vi "XW_Analysis_PN.vi"() -> (5 "Plug in titles":string[](array[string]), 7 "Plug in values":string[](array[string]))   [LabVIEW 2010]
uses:
  Controls/Save_Data.ctl
  Globals/Meas_global.vi
  Globals/Constants_global.vi
  Globals/Plug_in_data_global.vi
  <vilib>/Analysis/2dsp.llb/1D Auto Correlation (DBL).vi
  <vilib>/Analysis/2dsp.llb/1D Cross Correlation (DBL).vi
  Globals/Dynamic_call_global.ph.vi
  Controls/Inst_type.ctl
  <vilib>/Analysis/NI_AALPro.lvlib
panel:
  in  "Base output dir.":path=path "E:/TEST DUMP/QA test"
  in  "Instr. trav. pos index":i32=1 caption="Max moment order (n)"
  out "2nd comp.":string="v"
  out "DWT V":dbl[][](array[numeric])
  out "DWT U":dbl[][](array[numeric])
  out "Moment labels":string="u2\tu3\tu4\tv2\tv3\tv4\tu1v1\tu1v2\tu1v3\tu2v1\tu2v2\tu2v3\tu3v1\tu3v2\tu3v3\t"
  out "Moments":dbl[](array[numeric])=[1722182.8833231796, -3886.3484720409974, 2673329.388548149, 486662.5789464589, 30099.864061399367, 267894.77768629417, -362874.60480439797, -27342.46465798058, -171575.27046364895, 45307.846153853105, 346204.8570758366, 46417.28583948715, -555849.2877538406, -57883.486515684475, -276668.57969799754]
  in  "Max moment order (n)":i32=4
  in  "Psi pull-out search strings":string[](array[string])=["Psi 1:Average:Deg", "Psi 2:Average:Deg", "Psi 1:Max:Deg", "Psi 1:Min:Deg", "Psi 2:Max:Deg", "Psi 2:Min:Deg"]
  out "PwrSpec of UV":dbl[](array[numeric])
  out "AutoCovariance of UV":dbl[](array[numeric])
  out "Stats":dbl[][](array[numeric])=[[6.575279786237041, 9.737852813428246, 3.6304504106485544], [-0.05245759359759979, 2.477699101876975, -2.6510166405627658], [-0.4658815564167448, 17.436881271482232, -18.021292714723874]]
  in  "Use existing temp. block files":bool
  out "1D PDF UV":dbl[](array[numeric])=[0.0006999999999999999, 0.0012000000000000001, 0.0023, 0.009600000000000001, 0.021700000000000004, 0.04720000000000004, 0.1258000000000002, 0.3432, 0.8350999999999993, 1.9702000000000002, 4.395100000000001, 9.119700000000003, 17.268799999999995, 28.958799999999968, 41.936999999999976, 50.98729999999999, 50.53780000000002, 40.73420000000001, 26.46519999999999, 14.681399999999996, 6.8766, 2.8771999999999998, 1.1358999999999995, 0.4279000000000001, 0.14960000000000012, 0.055700000000000034, 0.021399999999999995, 0.008799999999999999, 0.0029000000000000007, 0.0009000000000000001, 0.0005, 0.0002]
  out "Axis UV":dbl[](array[numeric])=[-17.001377181562503, -15.8933092446875, -14.785241307812502, -13.677173370937501, -12.569105434062502, -11.461037497187501, -10.352969560312502, -9.244901623437501, -8.136833686562502, -7.028765749687502, -5.920697812812501, -4.8126298759375015, -3.7045619390625024, -2.5964940021875025, -1.4884260653125017, -0.3803581284375017, 0.7277098084374973, 1.8357777453124964, 2.943845682187497, 4.051913619062498, 5.159981555937497, 6.268049492812498, 7.376117429687499, 8.484185366562498, 9.592253303437497, 10.700321240312496, 11.808389177187497, 12.916457114062498, 14.024525050937497, 15.132592987812497, 16.240660924687496, 17.348728861562495] format="%0.2f"
  out "CrossPhaseSpec":dbl[](array[numeric])
  out "CrossPwrSpec":dbl[](array[numeric])
  out "df XPS":dbl=2.0 format="%0.2f"
  out "df APS":dbl=2.0 format="%0.2f"
  out "PwrSpec of U":dbl[](array[numeric])
  out "PwrSpec of V":dbl[](array[numeric])
  out "1D PDF V":dbl[](array[numeric])=[0.0002, 0.0002, 0.0007, 0.0023, 0.007300000000000003, 0.020099999999999996, 0.051100000000000007, 0.1565000000000002, 0.4621, 1.290799999999999, 3.148200000000002, 7.410600000000004, 15.145800000000001, 26.785999999999987, 39.79410000000002, 48.68330000000001, 48.59359999999999, 40.41779999999998, 28.99750000000001, 18.314799999999995, 10.619500000000002, 5.535599999999994, 2.625100000000002, 1.1498999999999997, 0.4730000000000003, 0.19190000000000013, 0.07570000000000006, 0.02819999999999999, 0.012799999999999997, 0.0037999999999999996, 0.0011, 0.00039999999999999996]
  out "Axis V":dbl[](array[numeric])=[-2.5184228665625, -2.3581504996875, -2.1978781328125, -2.0376057659375, -1.8773333990624999, -1.7170610321875, -1.5567886653124998, -1.3965162984375, -1.2362439315624998, -1.0759715646874999, -0.9156991978124999, -0.7554268309374998, -0.5951544640624997, -0.4348820971874998, -0.2746097303124999, -0.11433736343749978, 0.045935003437500344, 0.20620737031250047, 0.3664797371875004, 0.5267521040625003, 0.6870244709375004, 0.8472968378125003, 1.0075692046875002, 1.1678415715625003, 1.3281139384375003, 1.4883863053125004, 1.6486586721875005, 1.8089310390625002, 1.9692034059375003, 2.1294757728125004, 2.2897481396875006, 2.4500205065625007] format="%0.2f"
  out "Axis U":dbl[](array[numeric])=[-2.8494012174999996, -2.6585448925, -2.4676885674999998, -2.2768322425, -2.0859759175, -1.8951195925, -1.7042632674999998, -1.5134069424999999, -1.3225506175, -1.1316942925, -0.9408379675, -0.7499816424999999, -0.5591253174999997, -0.3682689924999998, -0.17741266749999984, 0.013443657500000095, 0.20429998250000003, 0.39515630749999997, 0.5860126324999999, 0.7768689574999998, 0.9677252825, 1.1585816075, 1.3494379324999999, 1.5402942575000003, 1.7311505825000002, 1.9220069075000001, 2.1128632325, 2.3037195575, 2.4945758825, 2.6854322075, 2.8762885325, 3.0671448574999998] format="%0.2f"
  out "1D PDF U":dbl[](array[numeric])=[0.0013000000000000002, 0.013600000000000001, 0.05110000000000003, 0.17249999999999993, 0.5014000000000004, 1.1012999999999988, 2.3825999999999983, 4.467200000000003, 7.386500000000001, 10.810400000000008, 14.8375, 19.03289999999999, 22.8511, 25.997799999999998, 27.798999999999992, 28.409600000000005, 27.990199999999987, 25.913499999999978, 22.712899999999976, 18.6365, 14.244500000000011, 10.149700000000005, 6.762300000000002, 3.9479000000000006, 2.1491000000000002, 1.0349999999999995, 0.39960000000000007, 0.16249999999999995, 0.04880000000000002, 0.0188, 0.012000000000000002, 0.0009]
  in  "XCovar algorithm":enum32{"direct", "frequency domain"}(ring)=enum."frequency domain"
  out "CrossCovariance":dbl[](array[numeric])
  in  "Non-dimensionalise covariance / spectra":bool=TRUE
  in  "Covariance normalisation":enum32{"none", "unbiased", "biased"}(ring)
  out "AutoCovariance of V":dbl[](array[numeric])
  out "AutoCovariance of U":dbl[](array[numeric])
  out "Post-Proc Block No.":i32=300
  in  "Interactive graph":bool
  in  "Mean shift PDFs":bool=TRUE
  in  "Nbins V":i32=32
  in  "Nbins U":i32=32
  in  "PDF (T) or Hist (F)":bool=TRUE
  out "VbinWidth":dbl=5.1287157400000005
  out "UbinWidth":dbl=6.1074024
  out "V bin centre vals.":dbl[](array[numeric])=[-0.03420117999999972]
  out "U bin centre vals.":dbl[](array[numeric])=[0.10887182000000006]
  out "2D PDF":dbl[][](array[numeric])=[[0.031925288878877155]]
  out "Quadrant probability":dbl[](array[numeric])=[0.18550766666666668, 0.31311866666666643, 0.3267083333333332, 0.17466533333333317]
  in  "Analysis":i32[](listbox)=[0, 1, 2, 4, 5, 6, 7]
  in  "format string":string="%.16f"
  in  "Instr. indices":i32[](array[numeric])=[1, 2]
  in  "Mode":enum16{"Spectra", "Autocorrelation"}(ring)
  in  "Separation Character":string="\t"
  in  "Precision":i16=16
  out "Ch names":string[](array[string])
  out "Output Directory":path=path "E:/TEST DUMP/QA test"
  in  "File":T1=enum."Save Data"
  # "You must have just these two indicators on the connector pane of the vi"
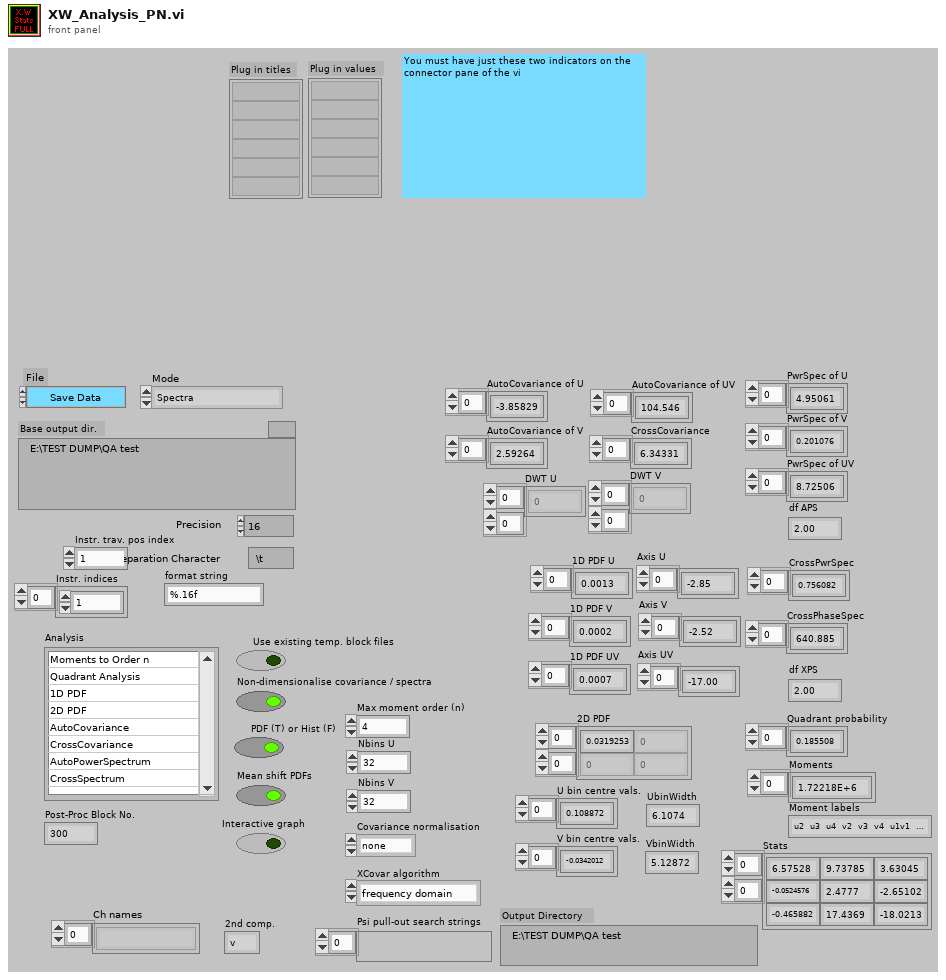
[diagram p1: front panel]
types:
  T1 = typedef "Save_Data.ctl" = enum16{"Save No Data", "Save Data"}
  T2 = typedef "Inst_type.ctl" = enum16{"Propeller anemometer", "Raw voltage", "Pressure Transducer", "Pitot-static tube", "Preston tube", "Hot wire", "Cross wire 1", "Cross wire 2", "Generic Linear", "Generic Polynomial", "Generic BackPoly", "Fast FID", "Thermocouple", "Cold wire", "Pulsed Wire", "LDA Vel", "LDA Tran time", "LDA Arr time"}
  T3 = enum32{"existing file", "new file", "new or existing file", "existing dir", "new dir", "new or existing dir", "existing file (use LLBs)", "new file (use LLBs)", "new or existing file (use LLBs)", "new or existing file or directory (use LLBs)"}
  T4 = cluster{"Name":string, "X":dbl, "Y":dbl, "Z":dbl}[]
  T5 = cluster{"Name":string, "X":dbl, "Y":dbl, "Z":dbl}
  T6 = typedef "Analysis_info_cluster.ctl" = cluster{"Colour":u32, "Inst type":T2, "Inst name":string, "Symbol":string, "Code name":string, "Extra Info":string, "Inst Array":T7, "Index":i32, "Voltage Index":i32, "Extra Titles":string[], "Extra Values":string[]}
  T7 = typedef "Instrument_Array.ctl" = enum16{"PWA", "LDA", "Analogue"}
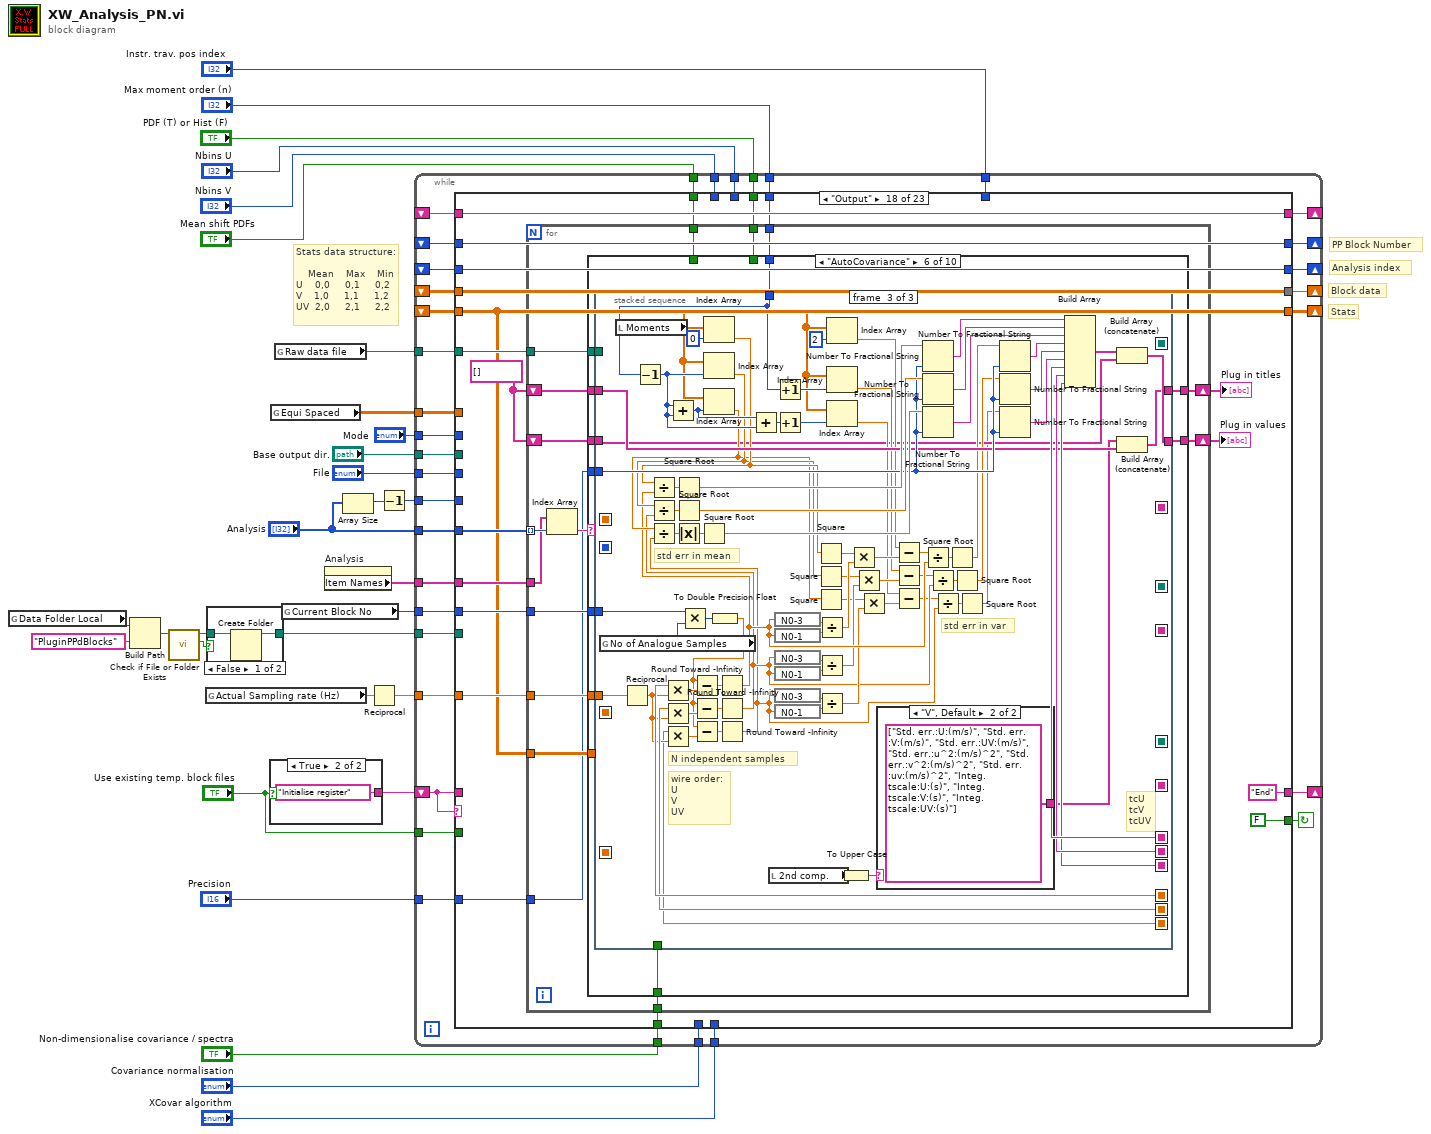
[diagram p0: block diagram]
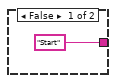
[diagram p3: hidden frame]
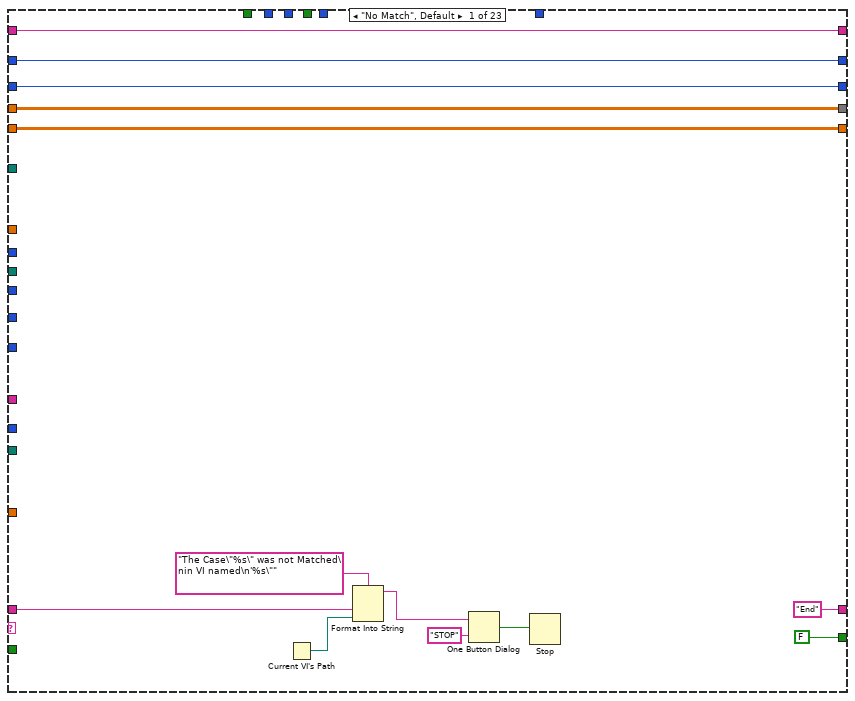
[diagram p4: hidden frame]
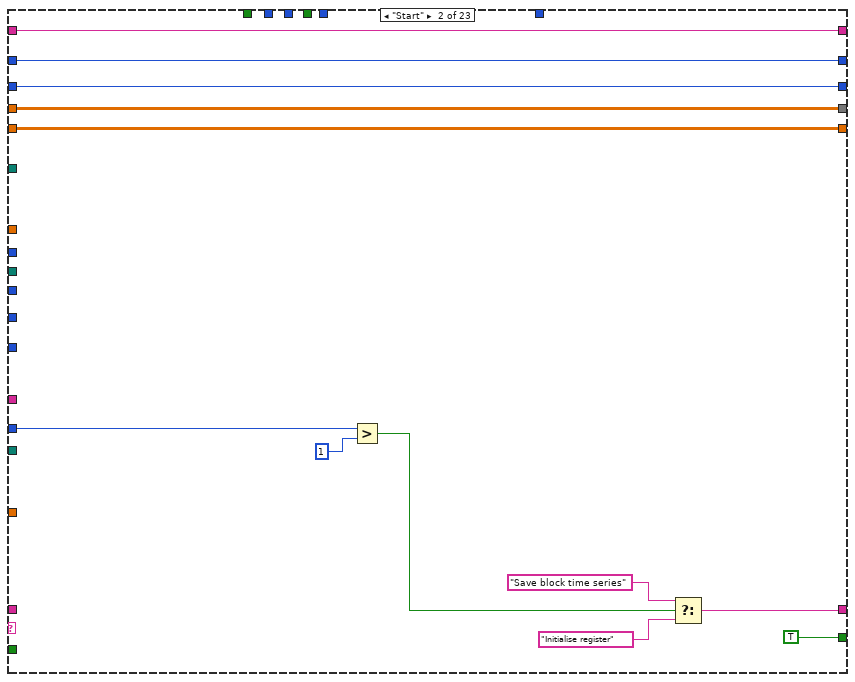
[diagram p5: hidden frame]
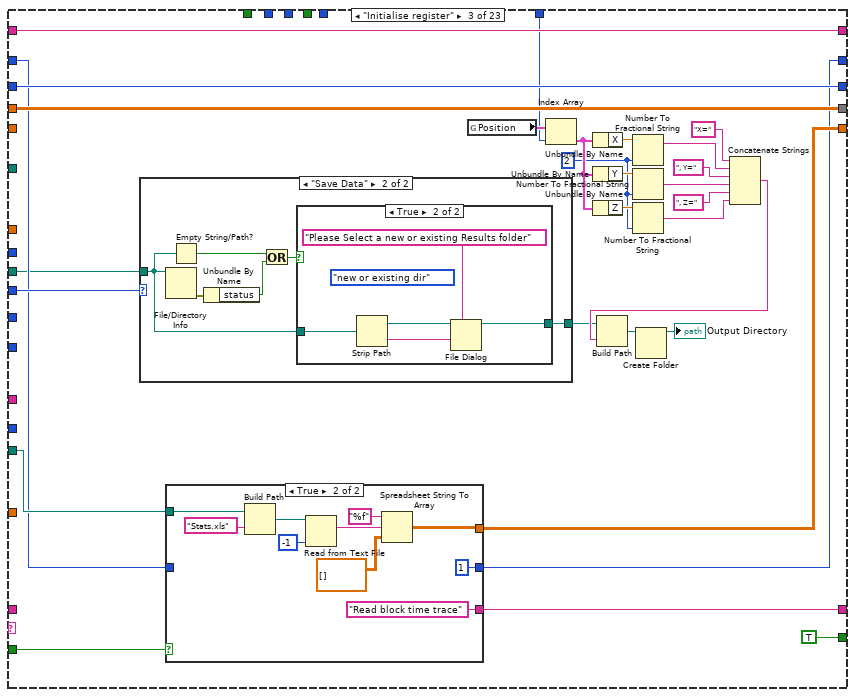
[diagram p6: hidden frame]
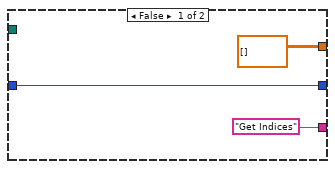
[diagram p7: hidden frame]
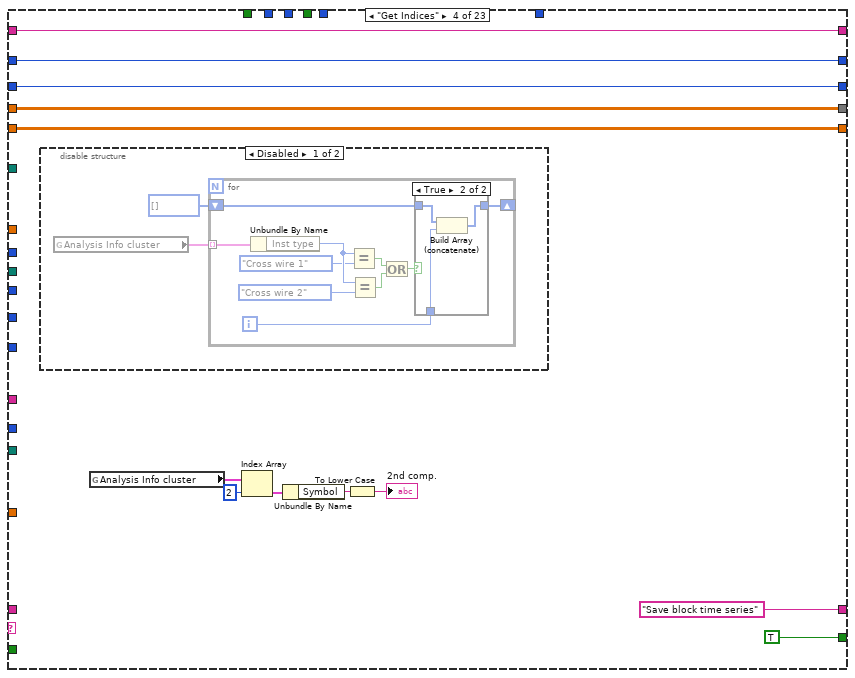
[diagram p10: hidden frame]
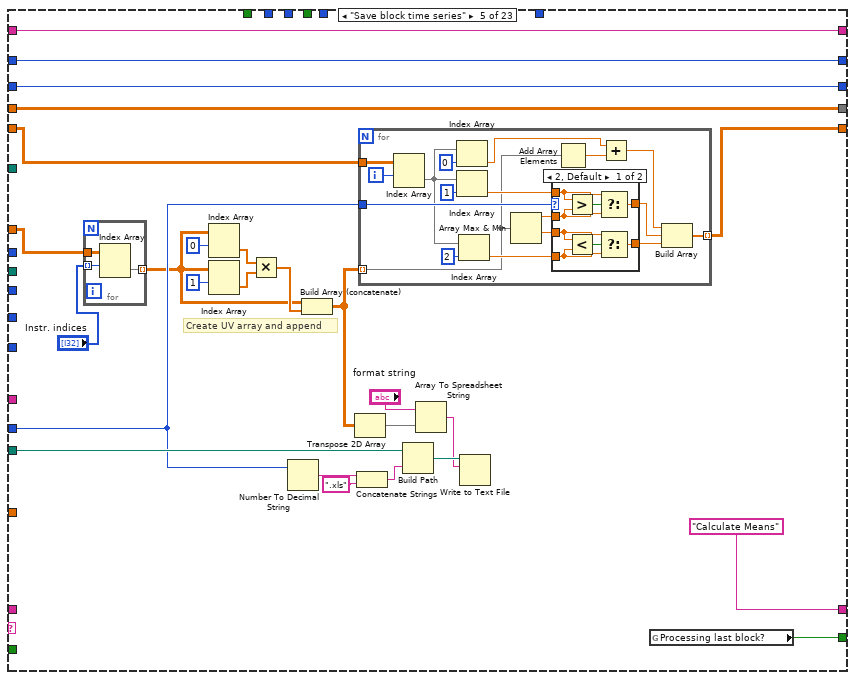
[diagram p13: hidden frame]
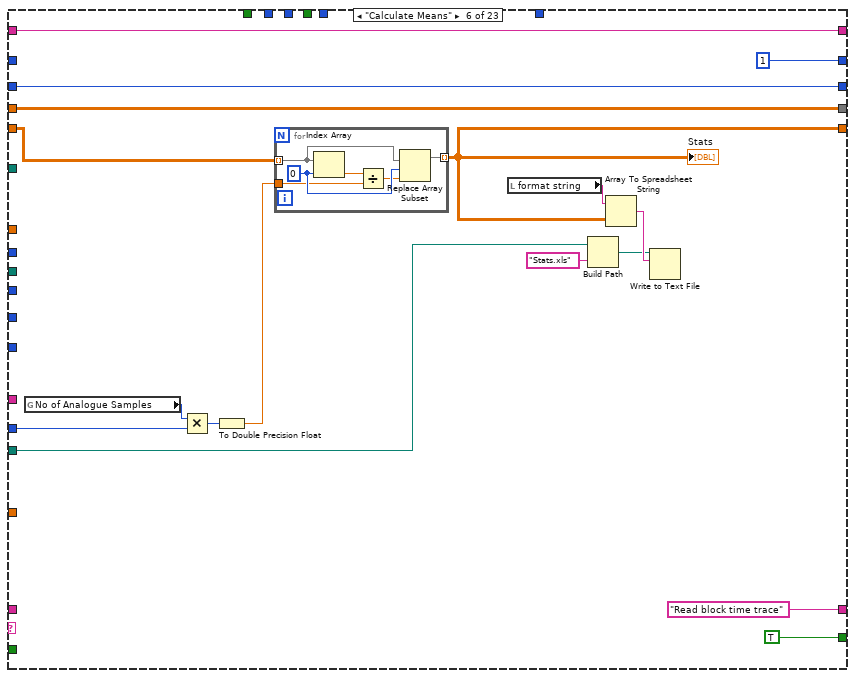
[diagram p15: hidden frame]
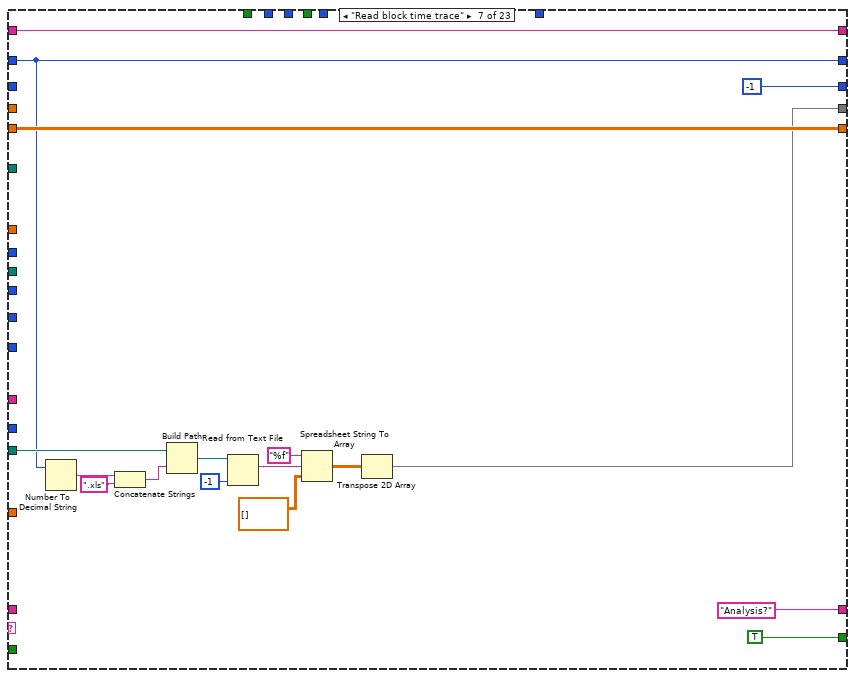
[diagram p16: hidden frame]
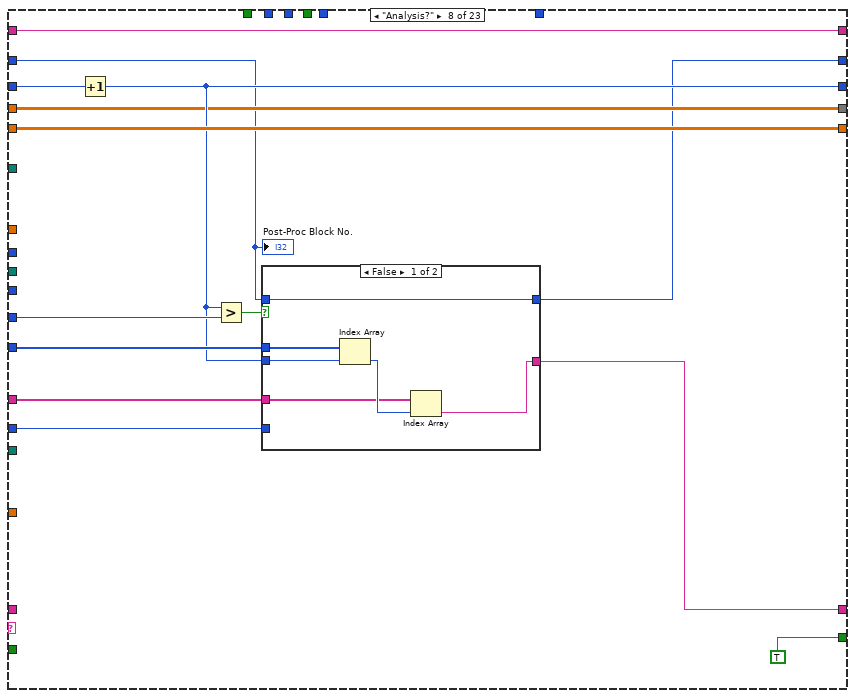
[diagram p17: hidden frame]
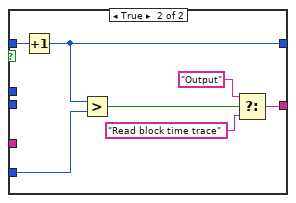
[diagram p18: hidden frame]
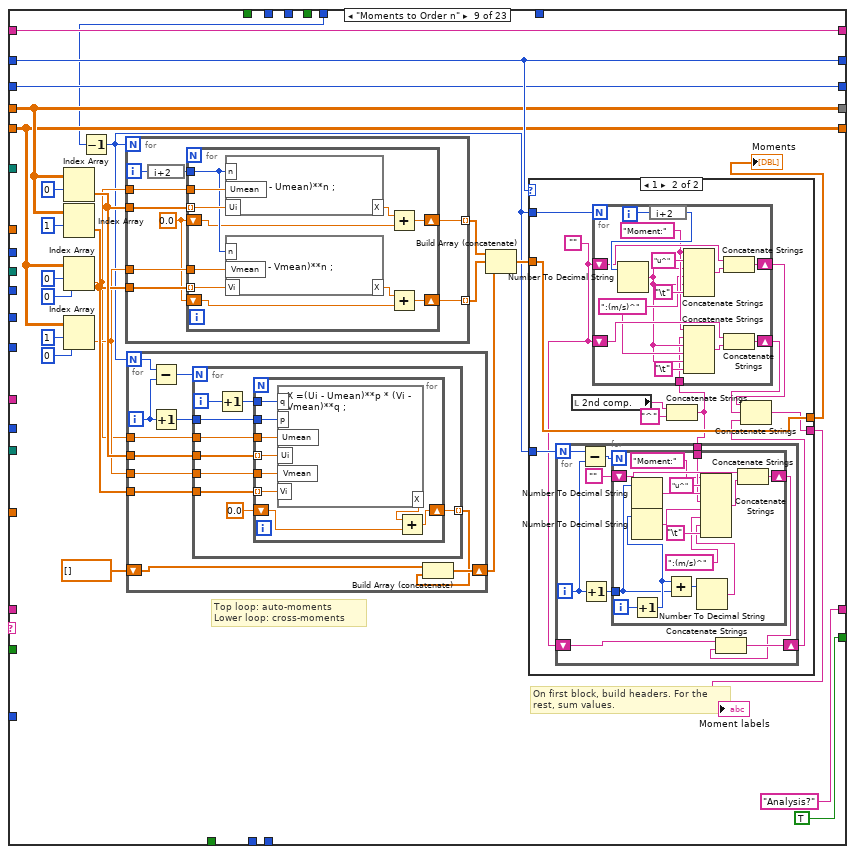
[diagram p19: hidden frame]
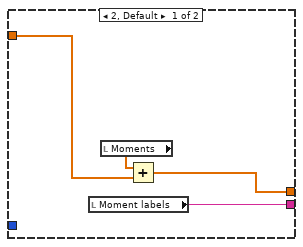
[diagram p20: hidden frame]
diagram:
  # "Stats data structure:\n\n    Mean    Max    Min\nU    0,0     0,1     0,2\nV    1,0     1,1     1,2\nUV  2,0     2,1     2,2"
  # "Analysis index"
  # "PP Block Number"
  # "Stats"
  # "Block data"
  n1 = global read "Constants_global.vi" "Data Folder Local"() -> (w27:path)
  n2 = Build Path(base path=w27, name or relative path="PluginPPdBlocks") -> (appended path=w6:path)
  n3 = call <vilib>:"Check if File or Folder Exists.vi"("path"=w6) -> ("file or folder exists?"=w5:bool, "dup path"=w4:path)  [unwired: 1 in, 8 out]
  n4 = global read "Meas_global.vi" "Actual Sampling rate (Hz)"() -> (w12:dbl)
  n5 = case shown="False" w5 {
    tunnel: w4 -> [w32 w33]
    tunnel: [w31 w33] -> w3
    frame False {
      n6 = Create Folder(path (use dialog)=w32) -> (created path=w31:path)  [unwired: 1 in, 3 out]
    }
    frame True {
    }
  }
  n7 = case shown="True" "Use existing temp. block files" {
    tunnel: ["Start" "Initialise register"] -> w9
    frame False {
    }
    frame True {
    }
  }
  n8 = global read "Plug_in_data_global.vi" "Equi Spaced"() -> (w30:dbl[][])
  n9 = global read "Meas_global.vi" "Raw data file"() -> (w25:path)
  n10 = global read "Meas_global.vi" "Current Block No"() -> (w29:i32)
  n11 = property on="Analysis" class="LstBox (strict)"() -> ("Item Names"=w23:string[])  [unwired: 2 in, 2 out]
  n12 = Array Size(array="Analysis") -> (size(s)=w21:i32)
  n13 = Reciprocal(x=w12) -> (1/x=w11:dbl)
  n14 = Decrement(x=w21) -> (x-1=w20:i32)
  n15 = while {
    shift-left: w9 -> [w70]
    shift-right: [w68] -> _
    tunnel: w30 -> [w69]
    shift-right: [w66] -> _
    shift-left: _ -> [w65]
    shift-right: [w64] -> _
    shift-left: _ -> [w63]
    tunnel: w29 -> [w62]
    tunnel: w3 -> [w61]
    shift-right: [w60] -> _
    shift-left: _ -> [w59]
    tunnel: "File" -> [w58]
    shift-right: [w57] -> _
    shift-left: _ -> [w56]
    tunnel: w25 -> [w55]
    shift-right: [w54] -> _
    shift-left: _ -> [w53]
    tunnel: "Mode" -> [w52]
    tunnel: "Analysis" -> [w51]
    tunnel: w23 -> [w50]
    tunnel: w20 -> [w49]
    tunnel: "PDF (T) or Hist (F)" -> [w48]
    tunnel: "Nbins U" -> [w47]
    tunnel: "Nbins V" -> [w46]
    tunnel: "Mean shift PDFs" -> [w45]
    tunnel: "Covariance normalisation" -> [w44]
    tunnel: "Non-dimensionalise covariance / spectra" -> [w43]
    tunnel: "XCovar algorithm" -> [w42]
    tunnel: w11 -> [w41]
    tunnel: "Use existing temp. block files" -> [w40]
    tunnel: "Precision" -> [w39]
    tunnel: "Max moment order (n)" -> [w38]
    tunnel: "Instr. trav. pos index" -> [w37]
    tunnel: "Base output dir." -> [w36]
    stop <- w67 continue-if-true
    n16 = case shown="\"Output\"" w70 {
      tunnel: ["End" ("t") w90 w118 "Save block time series" ("t") "Calculate Means" ("t") "Read block time trace" ("t") "Analysis?" ("t") w283 "Analysis?" ("t") "Analysis?" ("t") "Analysis?" ("t") "Analysis?" ("t") "Analysis?" ("t") "Analysis?" ("t") "Analysis?" ("t") "Analysis?" ("t") "Analysis?" ("t") "End" ("t") "Full Header info" ("t") "Add column titles" ("t") "Create Columns" ("t") "Save to file" ("t") "End" ("t")] -> w68
      tunnel: w70 -> [w79 _ _ _ _ _ _ _ _ _ _ _ _ _ _ _ _ _ _ _ _ _ _]
      tunnel: w69 -> [_ _ _ _ w181 _ _ _ _ _ _ _ _ _ _ _ _ _ _ _ _ _ _]
      tunnel: [FALSE TRUE TRUE ("Processing last block?") TRUE ("Processing last block?") w202 TRUE ("Processing last block?") TRUE ("Processing last block?") TRUE ("Processing last block?") TRUE TRUE TRUE TRUE TRUE TRUE TRUE TRUE TRUE FALSE TRUE ("Processing last block?") TRUE ("Processing last block?") TRUE ("Processing last block?") TRUE ("Processing last block?") FALSE] -> w67
      tunnel: [w76 w86 w117 w156 w196 w237 w273 w287 w313 w432 w475 w584 w628 w672 w694 w746 w779 w802 w1490 w1514 w1538 w1557 w1597] -> w66
      tunnel: w65 -> [w76 w86 _ w156 w194 w247 w273 w287 w313 w432 w475 w584 w628 w672 w694 w746 w779 w802 w1490 w1514 w1538 w1557 w1597]
      tunnel: [w74 w89 w121 w159 w197 w250 w260 w279 w324 w436 w483 w604 w625 w676 w697 w750 w782 w809 w1491 w1515 w1539 w1552 w1611] -> w64
      tunnel: w63 -> [w74 w89 w121 w159 w197 w250 _ w279 w324 w436 w483 w604 w625 w676 w697 w750 w782 w809 w1491 w1515 w1539 w1552 w1611]
      tunnel: w62 -> [_ w88 _ _ w195 w248 _ w276 _ w439 _ w597 _ _ _ _ _ w806 _ _ _ _ _]
      tunnel: w61 -> [_ _ w116 _ w203 w236 w267 _ _ _ _ _ _ _ _ _ _ _ _ _ _ _ _]
      tunnel: [w75 w87 w123 w160 w201 w252 -1 w280 w321 w433 w520 w601 w640 w673 w712 w747 w780 w810 w1492 w1516 w1540 w1558 w1612] -> w60
      tunnel: w59 -> [w75 w87 w123 w160 w201 w252 _ w285 w321 w433 w520 w601 w640 w673 w712 w747 w780 w810 w1492 w1516 w1540 w1558 w1612]
      tunnel: w58 -> [_ _ w124 _ _ _ _ _ _ _ _ _ _ _ _ _ _ _ _ _ _ _ _]
      tunnel: [w73 w85 w114 w161 w200 1 w266 w278 w325 w437 w468 w605 w619 w669 w689 w736 w774 w811 w1493 w1517 w1541 w1566 w1610] -> w57
      tunnel: w56 -> [w73 w85 w115 w161 w200 _ w266 w277 w325 w437 w468 w605 w619 w669 w689 w736 w774 w811 w1493 w1517 w1541 w1566 w1610]
      tunnel: w55 -> [_ _ _ _ _ _ _ _ _ _ _ _ _ _ _ _ _ w807 w1494 w1507 _ _ w1609]
      tunnel: [w72 w84 w122 w162 w199 w251 w274 w288 w327 w450 w529 w612 w648 w683 w720 w757 w789 w812 w1489 w1506 w1534 w1562 w1601] -> w54
      tunnel: w53 -> [w72 w84 w122 w162 w199 w251 w274 w288 w327 w450 w529 w612 w648 w683 w720 w757 w789 w812 _ w1513 w1528 w1563 w1601]
      tunnel: w52 -> [_ _ _ _ _ _ _ _ _ _ _ _ _ _ _ _ _ _ _ _ w1531 _ w1598]
      tunnel: w51 -> [_ _ _ _ _ _ _ w286 _ _ _ _ _ _ _ _ _ w818 _ _ _ _ _]
      tunnel: w50 -> [_ _ _ _ _ _ _ w284 _ _ _ _ _ _ _ _ _ w817 _ _ _ _ _]
      tunnel: w49 -> [_ _ _ _ _ _ _ w282 _ _ _ _ _ _ _ _ _ _ _ _ _ _ _]
      tunnel: w48 -> [_ _ _ _ _ _ _ _ _ _ _ w576 _ _ _ _ _ w804 _ _ _ _ _]
      tunnel: w47 -> [_ _ _ _ _ _ _ _ _ _ w471 w575 _ _ _ _ _ _ _ _ _ _ _]
      tunnel: w46 -> [_ _ _ _ _ _ _ _ _ _ w470 w574 _ _ _ _ _ _ _ _ _ _ _]
      tunnel: w45 -> [_ _ _ _ _ _ _ _ _ _ w498 w573 _ _ _ _ _ w801 _ _ _ _ _]
      tunnel: w44 -> [_ _ _ _ _ _ _ _ _ _ _ _ w620 w663 _ _ _ _ _ _ _ _ _]
      tunnel: w43 -> [_ _ _ _ _ _ _ _ _ _ _ _ _ _ _ _ _ w805 _ _ _ _ _]
      tunnel: w42 -> [_ _ _ _ _ _ _ _ _ _ _ _ _ w662 _ _ _ _ _ _ _ _ _]
      tunnel: w41 -> [_ _ _ _ _ _ _ _ _ _ _ _ _ _ w690 w739 w769 w803 _ _ _ _ _]
      tunnel: w40 -> [_ _ w119 _ _ _ _ _ _ _ _ _ _ _ _ _ _ _ _ _ _ _ _]
      tunnel: w39 -> [_ _ _ _ _ _ _ _ _ _ _ _ _ _ _ _ _ w800 _ _ _ w1551 _]
      tunnel: w38 -> [_ _ _ _ _ _ _ _ w304 _ _ _ _ _ _ _ _ w799 _ _ _ _ _]
      tunnel: w37 -> [_ _ w112 _ _ _ _ _ _ _ _ _ _ _ _ _ _ _ _ _ _ _ _]
      tunnel: w36 -> [_ _ w97 _ _ _ _ _ _ _ _ _ _ _ _ _ _ _ _ _ _ _ _]
      frame "No Match", Default {
        n17 = Current VI's Path() -> (path=w78:path)
        n18 = Format Into String(format string="The Case\"%s\" was not Matched\nin VI named\n'%s\"" ("Format String"), w79, w78) -> (resulting string=w82:string)  [unwired: 2 in, 1 out]
        n19 = One Button Dialog(message=w82, button name ("OK")="STOP") -> (true=w80:bool)
        n20 = Stop(stop? (T)=w80) -> ()
      }
      frame "Start" {
        n21 = Greater?(x=w88, y=1) -> (0:w92:bool)
        n22 = Select(t="Save block time series", s=w92, f="Initialise register") -> (s? t:f=w90:string)
      }
      frame "Initialise register" {
        w98 = i16 2 ("precision (6)")
        n23 = case shown="\"Save Data\"" w124 {
          tunnel: w97 -> [w138 w143]
          tunnel: [w138 w139] -> w100
          frame "Save No Data" {
          }
          frame "Save Data" {
            n24 = File/Directory Info(path=w143) -> (error out=w144:errorcluster)  [unwired: 1 in, 6 out]
            n25 = Empty String/Path?(string/path=w143) -> (empty?=w141:bool)
            n26 = Unbundle By Name(w144) -> ("status"=w142:bool)
            n27 = Or(x=w141, y=w142) -> (x .or. y?=w140:bool)
            n28 = case shown="True" w140 {
              tunnel: [w145 w150] -> w139
              tunnel: w143 -> [w145 w148]
              frame False {
              }
              frame True {
                (unwired) T3."new or existing dir" ("select mode (2)")
                n29 = Strip Path(path=w148) -> (stripped path=w147:path, name=w146:string)
                n30 = File Dialog(7:"Please Select a new or existing Results folder" ("prompt"), 9:w146, 11:w147) -> (3:w150:path)  [unwired: 1 in, 6 out]
              }
            }
          }
        }
        n31 = case shown="True" w119 {
          tunnel: ["Get Indices" ("t") "Read block time trace" ("t")] -> w118
          tunnel: [dbl[][] [] w129] -> w117
          tunnel: w116 -> [_ w131]
          tunnel: w115 -> [w125 _]
          tunnel: [w125 1 ("count")] -> w114
          frame False {
          }
          frame True {
            n32 = Build Path(base path=w131, name or relative path="Stats.xls") -> (appended path=w135:path)
            n33 = Read from Text File(file (use dialog)=w135, count=-1) -> (text=w133:string)  [unwired: 1 in, 4 out]
            n34 = Spreadsheet String To Array(format string="%f", spreadsheet string=w133, array type (2D Dbl)=dbl[][] []) -> (array=w129:dbl[][])  [unwired: 1 out]
          }
        }
        n35 = global read "Meas_global.vi" "Position"() -> (w113:T4)
        n36 = Index Array(array=w113, index=w112) -> (element=w111:T5)
        n37 = Unbundle By Name(w111) -> ("X"=w107:dbl)
        n38 = Unbundle By Name(w111) -> ("Y"=w105:dbl)
        n39 = Unbundle By Name(w111) -> ("Z"=w103:dbl)
        n40 = Number To Fractional String(number=w107, precision (6)=w98) -> (F-format string=w106:string)  [unwired: 2 out]
        n41 = Number To Fractional String(number=w105, precision (6)=w98) -> (F-format string=w104:string)  [unwired: 2 out]
        n42 = Number To Fractional String(number=w103, precision (6)=w98) -> (F-format string=w102:string)  [unwired: 2 out]
        n43 = Concatenate Strings("X=" ("string"), w106, ", Y=" ("string"), w104, ", Z=" ("string"), w102) -> (w101:string)
        n44 = Build Path(base path=w100, name or relative path=w101) -> (appended path=w99:path)
        n45 = Create Folder(path (use dialog)=w99) -> (created path=→"Output Directory":path)  [unwired: 1 in, 3 out]
      }
      frame "Get Indices" {
        n46 = disable-structure shown="Disabled" {
          frame Disabled {
            n47 = global read "Meas_global.vi" "Analysis Info cluster"() -> (w164:T6[])
            n48 = for {
              tunnel: w164 -> [w165] mode=indexing
              shift-right: [w166] -> _
              shift-left: i32[] [] -> [w168]
              i -> [w167]
              n49 = Unbundle By Name(w165) -> ("Inst type"=w174:T2)
              n50 = Equal?(x=w174, y=Inst_type."Cross wire 1" ("Inst type")) -> (x = y?=w171:bool)
              n51 = Equal?(x=w174, y=Inst_type."Cross wire 2" ("Inst type")) -> (x = y?=w170:bool)
              n52 = Or(x=w171, y=w170) -> (x .or. y?=w169:bool)
              n53 = case shown="True" w169 {
                tunnel: w168 -> [w175 w178]
                tunnel: w167 -> [_ w177]
                tunnel: [w175 w176] -> w166
                frame False {
                }
                frame True {
                  n54 = Build Array (concatenate)(w178, w177) -> (w176:i32[])
                }
              }
            }
          }
          frame Enabled {
          }
        }
        n55 = global read "Meas_global.vi" "Analysis Info cluster"() -> (w155:T6[])
        n56 = Index Array(array=w155, index=2) -> (element=w154:T6)
        n57 = Unbundle By Name(w154) -> ("Symbol"=w152:string)
        n58 = To Lower Case(string=w152) -> (all lower case string=→"2nd comp.":string)
      }
      frame "Save block time series" {
        # "Create UV array and append"
        n59 = for {
          tunnel: "Instr. indices" -> [w207] mode=indexing
          tunnel: w181 -> [w206]
          tunnel: [w205] -> w183 mode=indexing
          n60 = Index Array(array=w206, index (row)=w207) -> (element=w205:dbl[])  [unwired: 1 in]
        }
        n61 = Index Array(array=w183, index (row)=0 ("index")) -> (element=w191:dbl[])  [unwired: 1 in]
        n62 = Index Array(array=w183, index (row)=1 ("index")) -> (element=w190:dbl[])  [unwired: 1 in]
        n63 = Multiply(x=w191, y=w190) -> (x*y=w189:dbl[])
        n64 = Number To Decimal String(number=w195) -> (decimal integer string=w188:string)  [unwired: 1 out]
        n65 = Build Array (concatenate)(w183, w189) -> (w180:dbl[][])
        n66 = Transpose 2D Array(2D array=w180) -> (transposed array=w182:dbl[][])
        n67 = Concatenate Strings(w188, ".xls" ("string")) -> (w186:string)
        n68 = for {
          tunnel: w180 -> [w208] mode=indexing
          tunnel: [w222] -> w196 mode=indexing
          tunnel: w195 -> [w221]
          tunnel: w194 -> [w215]
          i -> [w216]
          n69 = Index Array(array=w215, index (row)=w216) -> (element=w213:dbl[])  [unwired: 1 in]
          n70 = Index Array(array=w213, index=0) -> (element=w210:dbl)
          n71 = Index Array(array=w213, index=1) -> (element=w218:dbl)
          n72 = Index Array(array=w213, index=2) -> (element=w217:dbl)
          n73 = Array Max & Min(array=w208) -> (max value=w225:dbl, min value=w224:dbl)  [unwired: 2 out]
          n74 = case shown="2, Default" w221 {
            tunnel: [w229 w235] -> w212
            tunnel: w225 -> [w232 w235]
            tunnel: [w228 w234] -> w223
            tunnel: w224 -> [w227 w234]
            tunnel: w218 -> [w230 _]
            tunnel: w217 -> [w226 _]
            frame 2, Default {
              n75 = Greater?(x=w230, y=w232) -> (0:w233:bool)
              n76 = Less?(x=w227, y=w226) -> (x < y?=w231:bool)
              n77 = Select(t=w230, s=w233, f=w232) -> (s? t:f=w229:dbl)
              n78 = Select(t=w227, s=w231, f=w226) -> (s? t:f=w228:dbl)
            }
            frame 1 {
            }
          }
          n79 = Add Array Elements(numeric array=w208) -> (sum=w209:dbl)
          n80 = Add(x=w210, y=w209) -> (x+y=w211:dbl)
          n81 = Build Array(w211, w212, w223) -> (w222:dbl[])
        }
        n82 = Build Path(base path=w203, name or relative path=w186) -> (appended path=w185:path)
        n83 = Array To Spreadsheet String(array=w182, 3:"format string") -> (spreadsheet string=w184:string)  [unwired: 1 out]
        n84 = Write to Text File(file (use dialog)=w185, text=w184) -> ()  [unwired: 1 in, 4 out]
        n85 = global read "Meas_global.vi" "Processing last block?"() -> (w202:bool)
      }
      frame "Calculate Means" {
        n86 = global read "Meas_global.vi" "No of Analogue Samples"() -> (w249:i32)
        n87 = Multiply(x=w249, y=w248) -> (x*y=w243:i32)
        n88 = To Double Precision Float(number=w243) -> (double precision float=w242:dbl)
        n89 = for {
          tunnel: w247 -> [w255] mode=indexing
          tunnel: [w254] -> w237 mode=indexing
          tunnel: w242 -> [w253]
          w257 = 0 ("index")
          n90 = Index Array(array=w255, index=w257) -> (element=w258:dbl)
          n91 = Divide(x=w258, y=w253) -> (x/y=w256:dbl)
          n92 = Replace Array Subset(array=w255, new element=w256, index=w257) -> (w254:dbl[])
        }
        "Stats" <- w237
        n93 = local read "format string"() -> (w239:string)
        n94 = Build Path(base path=w236, name or relative path="Stats.xls") -> (appended path=w238:path)
        n95 = Array To Spreadsheet String(array=w237, 3:w239) -> (spreadsheet string=w240:string)  [unwired: 1 out]
        n96 = Write to Text File(file (use dialog)=w238, text=w240) -> ()  [unwired: 1 in, 4 out]
      }
      frame "Read block time trace" {
        n97 = Number To Decimal String(number=w266) -> (decimal integer string=w270:string)  [unwired: 1 out]
        n98 = Concatenate Strings(w270, ".xls" ("string")) -> (w268:string)
        n99 = Build Path(base path=w267, name or relative path=w268) -> (appended path=w265:path)
        n100 = Read from Text File(file (use dialog)=w265, count=-1) -> (text=w263:string)  [unwired: 1 in, 4 out]
        n101 = Spreadsheet String To Array(format string="%f", spreadsheet string=w263, array type (2D Dbl)=dbl[][] []) -> (array=w261:dbl[][])  [unwired: 1 out]
        n102 = Transpose 2D Array(2D array=w261) -> (transposed array=w260:dbl[][])
      }
      frame "Analysis?" {
        n103 = Increment(x=w285) -> (x+1=w280:i32)
        n104 = Greater?(x=w280, y=w282) -> (0:w281:bool)
        n105 = case shown="False" w281 {
          tunnel: w286 -> [w295 _]
          tunnel: w284 -> [w293 _]
          tunnel: [w292 w298] -> w283
          tunnel: w280 -> [w291 _]
          tunnel: w277 -> [w290 w302]
          tunnel: w276 -> [_ w301]
          tunnel: [w290 w296] -> w278
          frame False {
            n106 = Index Array(array=w295, index=w291) -> (element=w294:i32)
            n107 = Index Array(array=w293, index=w294) -> (element=w292:string)
          }
          frame True {
            n108 = Increment(x=w302) -> (x+1=w296:i32)
            n109 = Greater?(x=w296, y=w301) -> (0:w300:bool)
            n110 = Select(t="Output", s=w300, f="Read block time trace") -> (s? t:f=w298:string)
          }
        }
        "Post-Proc Block No." <- w277
      }
      frame "Moments to Order n" {
        # "On first block, build headers. For the\nrest, sum values."
        # "Top loop: auto-moments\nLower loop: cross-moments"
        n111 = Index Array(array=w324, index (row)=0) -> (element=w310:dbl[])  [unwired: 1 in]
        n112 = Index Array(array=w324, index (row)=1) -> (element=w309:dbl[])  [unwired: 1 in]
        n113 = Index Array(array=w313, index (row)=0, index (col)=0 ("disabled index (col)")) -> (element=w307:dbl)
        n114 = Index Array(array=w313, index (row)=1, index (col)=0 ("disabled index (col)")) -> (element=w308:dbl)
        n115 = Decrement(x=w304) -> (x-1=w303:i32)
        n116 = for {
          N: w303 -> [_]
          tunnel: w307 -> [w366]
          tunnel: w310 -> [w365]
          tunnel: w309 -> [w364]
          tunnel: w308 -> [w363]
          tunnel: [w361] -> w312 mode=indexing
          tunnel: [w360] -> w311 mode=indexing
          i -> [w359]
          w362 = 0.0
          n117 = expression code="i+2"(w359) -> (w358:i32)
          n118 = for {
            tunnel: w366 -> [w377]
            tunnel: w365 -> [w376] mode=indexing
            shift-right: [w368] -> w361
            shift-left: w362 -> [w367]
            tunnel: w364 -> [w375] mode=indexing
            tunnel: w363 -> [w374]
            shift-right: [w369] -> w360
            shift-left: w362 -> [w370]
            tunnel: w358 -> [w373]
            n119 = formula code="X =(Ui - Umean)**n ;"("Umean"=w377, "Ui"=w376, "n"=w373) -> ("X"=w372:dbl)
            n120 = formula code="X =(Vi - Vmean)**n ;"("Vmean"=w374, "Vi"=w375, "n"=w373) -> ("X"=w371:dbl)
            n121 = Add(x=w372, y=w367) -> (x+y=w368:dbl)
            n122 = Add(x=w371, y=w370) -> (x+y=w369:dbl)
          }
        }
        n123 = for {
          N: w303 -> [w330]
          tunnel: w310 -> [w339]
          tunnel: w309 -> [w338]
          tunnel: w308 -> [w337]
          tunnel: w307 -> [w336]
          shift-right: [w334] -> w305
          shift-left: dbl[] [] -> [w335]
          i -> [w331]
          n124 = Subtract(x=w330, y=w331) -> (x-y=w329:i32)
          n125 = Increment(x=w331) -> (x+1=w332:i32)
          n126 = for {
            N: w329 -> [_]
            tunnel: w336 -> [w348]
            tunnel: w339 -> [w347]
            tunnel: [w342] -> w333 mode=indexing
            tunnel: w337 -> [w345]
            tunnel: w338 -> [w344]
            tunnel: w332 -> [w343]
            i -> [w341]
            n127 = Increment(x=w341) -> (x+1=w340:i32)
            n128 = for {
              tunnel: w348 -> [w357]
              tunnel: w347 -> [w356] mode=indexing
              shift-right: [w354] -> w342
              shift-left: 0.0 -> [w353]
              tunnel: w340 -> [w350]
              tunnel: w345 -> [w352]
              tunnel: w344 -> [w351] mode=indexing
              tunnel: w343 -> [w349]
              n129 = formula code="X =(Ui - Umean)**p * (Vi - Vmean)**q ;"("Umean"=w357, "Ui"=w356, "p"=w349, "Vi"=w351, "Vmean"=w352, "q"=w350) -> ("X"=w355:dbl)
              n130 = Add(x=w355, y=w353) -> (x+y=w354:dbl)
            }
          }
          n131 = Build Array (concatenate)(w335, w333) -> (w334:dbl[])
        }
        n132 = Build Array (concatenate)(w312, w311, w305) -> (w319:dbl[])
        n133 = case shown="1" w325 {
          tunnel: [w381 w389] -> w323
          tunnel: w303 -> [_ w392]
          tunnel: [w379 w388] -> w320
          tunnel: w319 -> [w378 w389]
          tunnel: w303 -> [_ w387]
          frame 2, Default {
            n134 = local read "Moment labels"() -> (w379:string)
            n135 = local read "Moments"() -> (w380:dbl[])
            n136 = Add(x=w380, y=w378) -> (x+y=w381:dbl[])
          }
          frame 1 {
            w385 = ""
            n137 = local read "2nd comp."() -> (w383:string)
            n138 = Concatenate Strings(w383, "^" ("string")) -> (w382:string)
            n139 = for {
              N: w387 -> [w394]
              shift-right: [w400] -> w386
              shift-left: w385 -> [w399]
              tunnel: w382 -> [w396]
              i -> [w395]
              n140 = Subtract(x=w394, y=w395) -> (x-y=w393:i32)
              n141 = Increment(x=w395) -> (x+1=w401:i32)
              n142 = for {
                N: w393 -> [_]
                shift-right: [w414] -> w397
                shift-left: "" -> [w410]
                tunnel: w401 -> [w408]
                tunnel: w396 -> [w403]
                i -> [w411]
                n143 = Number To Decimal String(number=w408) -> (decimal integer string=w413:string)  [unwired: 1 out]
                n144 = Increment(x=w411) -> (x+1=w409:i32)
                n145 = Number To Decimal String(number=w409) -> (decimal integer string=w412:string)  [unwired: 1 out]
                n146 = Add(x=w409, y=w408) -> (x+y=w406:i32)
                n147 = Number To Decimal String(number=w406) -> (decimal integer string=w405:string)  [unwired: 1 out]
                n148 = Concatenate Strings("Moment:" ("t"), "u^" ("t"), w413, w403, w412, ":(m/s)^" ("t"), w405, "\t") -> (w415:string)
                n149 = Concatenate Strings(w410, w415) -> (w414:string)
              }
              n150 = Concatenate Strings(w399, w397) -> (w400:string)
            }
            n151 = for {
              N: w392 -> [_]
              shift-right: [w424] -> w391
              shift-left: w385 -> [w426]
              shift-right: [w423] -> w390
              shift-left: w385 -> [w425]
              tunnel: w382 -> [w417]
              i -> [w431]
              w419 = ":(m/s)^" ("t")
              w421 = "Moment:" ("t")
              n152 = expression code="i+2"(w431) -> (w427:i32)
              n153 = Number To Decimal String(number=w427) -> (decimal integer string=w418:string)  [unwired: 1 out]
              n154 = Concatenate Strings(w421, "u^" ("t"), w418, w419, w418, "\t") -> (w429:string)
              n155 = Concatenate Strings(w421, w417, w418, w419, w418, "\t") -> (w428:string)
              n156 = Concatenate Strings(w426, w429) -> (w424:string)
              n157 = Concatenate Strings(w425, w428) -> (w423:string)
            }
            n158 = Concatenate Strings(w391, w390, w386) -> (w388:string)
          }
        }
        "Moments" <- w323
        "Moment labels" <- w320
      }
      frame "Quadrant Analysis" {
        n159 = Index Array(array=w436, index (row)=1) -> (element=w446:dbl[])  [unwired: 1 in]
        n160 = Index Array(array=w432, index (row)=0, index (col)=0 ("disabled index (col)")) -> (element=w441:dbl)
        n161 = Index Array(array=w436, index (row)=0) -> (element=w447:dbl[])  [unwired: 1 in]
        n162 = Index Array(array=w432, index (row)=1, index (col)=0 ("disabled index (col)")) -> (element=w440:dbl)
        n163 = call "XW quadrant analysis, PN.vi"("V"=w446, "Umean"=w441, "Vmean"=w440, "No. of blocks"=w439, "U"=w447) -> ("Quadrant probability"=w438:dbl[])
        n164 = case shown="2, Default" w437 {
          tunnel: w438 -> [w453 w455]
          tunnel: [w454 w455] -> w435
          frame 2, Default {
            n165 = local read "Quadrant probability"() -> (w452:dbl[])
            n166 = Add(x=w452, y=w453) -> (x+y=w454:dbl[])
          }
          frame 1 {
          }
        }
        "Quadrant probability" <- w435
      }
      frame "1D PDF" {
        w472 = enum32{"lower", "upper"}."upper" ("inclusion")
        n167 = Index Array(array=w483, index (row)=0) -> (element=w497:dbl[])  [unwired: 1 in]
        n168 = Index Array(array=w483, index (row)=1) -> (element=w495:dbl[])  [unwired: 1 in]
        n169 = Index Array(array=w483, index (row)=2) -> (element=w482:dbl[])  [unwired: 1 in]
        n170 = Index Array(array=w475, index (row)=0, index (col)=1 ("disabled index (col)")) -> (element=w467:dbl)
        n171 = Index Array(array=w475, index (row)=0, index (col)=2 ("disabled index (col)")) -> (element=w466:dbl)
        n172 = Index Array(array=w475, index (row)=1, index (col)=1 ("disabled index (col)")) -> (element=w463:dbl)
        n173 = Index Array(array=w475, index (row)=1, index (col)=2 ("disabled index (col)")) -> (element=w462:dbl)
        n174 = Index Array(array=w475, index (row)=0, index (col)=0 ("disabled index (col)")) -> (element=w496:dbl)
        n175 = Index Array(array=w475, index (row)=1, index (col)=0 ("disabled index (col)")) -> (element=w494:dbl)
        n176 = Index Array(array=w475, index (row)=2, index (col)=0 ("disabled index (col)")) -> (element=w474:dbl)
        n177 = Index Array(array=w475, index (row)=2, index (col)=1 ("disabled index (col)")) -> (element=w459:dbl)
        n178 = Index Array(array=w475, index (row)=2, index (col)=2 ("disabled index (col)")) -> (element=w458:dbl)
        n179 = case shown="True" w498 {
          tunnel: w497 -> [w543 w564]
          tunnel: w496 -> [_ w556]
          tunnel: w495 -> [w542 w563]
          tunnel: w494 -> [_ w555]
          tunnel: [w543 w562] -> w493
          tunnel: [w542 w561] -> w492
          tunnel: [w541 w560] -> w473
          tunnel: w482 -> [w541 w559]
          tunnel: w474 -> [_ w554]
          tunnel: [w540 w558] -> w465
          tunnel: [w539 w557] -> w464
          tunnel: w467 -> [w540 w553]
          tunnel: w466 -> [w539 w552]
          tunnel: w463 -> [w538 w551]
          tunnel: w462 -> [w537 w550]
          tunnel: [w538 w549] -> w461
          tunnel: [w537 w548] -> w460
          tunnel: w459 -> [w536 w547]
          tunnel: w458 -> [w535 w546]
          tunnel: [w536 w545] -> w457
          tunnel: [w535 w544] -> w456
          frame False {
          }
          frame True {
            n180 = Subtract(x=w564, y=w556) -> (x-y=w562:dbl[])
            n181 = Subtract(x=w563, y=w555) -> (x-y=w561:dbl[])
            n182 = Subtract(x=w559, y=w554) -> (x-y=w560:dbl[])
            n183 = Subtract(x=w553, y=w556) -> (x-y=w558:dbl)
            n184 = Subtract(x=w552, y=w556) -> (x-y=w557:dbl)
            n185 = Subtract(x=w551, y=w555) -> (x-y=w549:dbl)
            n186 = Subtract(x=w550, y=w555) -> (x-y=w548:dbl)
            n187 = Subtract(x=w547, y=w554) -> (x-y=w545:dbl)
            n188 = Subtract(x=w546, y=w554) -> (x-y=w544:dbl)
          }
        }
        n189 = Max & Min(x=w471, y=w470) -> (min(x,y)=w469:i32)  [unwired: 1 out]
        n190 = call <vilib>:"General Histogram.vi"("X"=w493, "max"=w465, "min"=w464, "# bins"=w471, "inclusion"=w472) -> ("Histogram"=w513:i32[], "Axis"=→"Axis U":dbl[])  [unwired: 1 in, 8 out]
        n191 = call <vilib>:"General Histogram.vi"("X"=w492, "max"=w461, "min"=w460, "# bins"=w470, "inclusion"=w472) -> ("Histogram"=w504:i32[], "Axis"=→"Axis V":dbl[])  [unwired: 1 in, 8 out]
        n192 = call <vilib>:"General Histogram.vi"("X"=w473, "max"=w457, "min"=w456, "# bins"=w469, "inclusion"=w472) -> ("Histogram"=w490:i32[], "Axis"=→"Axis UV":dbl[])  [unwired: 1 in, 8 out]
        n193 = To Double Precision Float(number=w513) -> (double precision float=w512:dbl[])
        n194 = To Double Precision Float(number=w504) -> (double precision float=w506:dbl[])
        n195 = To Double Precision Float(number=w490) -> (double precision float=w488:dbl[])
        n196 = Array Size(array=w493) -> (size(s)=w511:i32)
        n197 = Array Size(array=w492) -> (size(s)=w507:i32)
        n198 = Array Size(array=w473) -> (size(s)=w487:i32)
        n199 = To Double Precision Float(number=w511) -> (double precision float=w510:dbl)
        n200 = To Double Precision Float(number=w507) -> (double precision float=w508:dbl)
        n201 = To Double Precision Float(number=w487) -> (double precision float=w486:dbl)
        n202 = Divide(x=w512, y=w510) -> (x/y=w509:dbl[])
        n203 = Divide(x=w506, y=w508) -> (x/y=w503:dbl[])
        n204 = Divide(x=w488, y=w486) -> (x/y=w491:dbl[])
        n205 = case shown="2, Default" w468 {
          tunnel: [w571 w572] -> w522
          tunnel: w509 -> [w569 w572]
          frame 2, Default {
            n206 = local read "1D PDF U"() -> (w570:dbl[])
            n207 = Add(x=w570, y=w569) -> (x+y=w571:dbl[])
          }
          frame 1 {
          }
        }
        "1D PDF U" <- w522
        n208 = case shown="2, Default" w468 {
          tunnel: [w567 w568] -> w514
          tunnel: w503 -> [w565 w568]
          frame 2, Default {
            n209 = local read "1D PDF V"() -> (w566:dbl[])
            n210 = Add(x=w566, y=w565) -> (x+y=w567:dbl[])
          }
          frame 1 {
          }
        }
        "1D PDF V" <- w514
        n211 = case shown="2, Default" w468 {
          tunnel: [w533 w534] -> w485
          tunnel: w491 -> [w531 w534]
          frame 2, Default {
            n212 = local read "1D PDF UV"() -> (w532:dbl[])
            n213 = Add(x=w532, y=w531) -> (x+y=w533:dbl[])
          }
          frame 1 {
          }
        }
        "1D PDF UV" <- w485
      }
      frame "2D PDF" {
        n214 = Index Array(array=w604, index (row)=0) -> (element=w599:dbl[])  [unwired: 1 in]
        n215 = Index Array(array=w604, index (row)=1) -> (element=w598:dbl[])  [unwired: 1 in]
        n216 = Index Array(array=w584, index (row)=0, index (col)=0 ("disabled index (col)")) -> (element=w596:dbl)
        n217 = Index Array(array=w584, index (row)=1, index (col)=0 ("disabled index (col)")) -> (element=w595:dbl)
        n218 = Index Array(array=w584, index (row)=0, index (col)=1 ("disabled index (col)")) -> (element=w590:dbl)
        n219 = Index Array(array=w584, index (row)=0, index (col)=2 ("disabled index (col)")) -> (element=w589:dbl)
        n220 = Index Array(array=w584, index (row)=1, index (col)=1 ("disabled index (col)")) -> (element=w583:dbl)
        n221 = Index Array(array=w584, index (row)=1, index (col)=2 ("disabled index (col)")) -> (element=w582:dbl)
        n222 = call "2D Histogram or PDF, PN.vi"("Nbins U"=w575, "Nbins V"=w574, "Mean shift"=w573, "Umean"=w596, "Vmean"=w595, "Umax"=w590, "No. of blocks"=w597, "Umin"=w589, "PDF"=w576, "Interactive graph"="Interactive graph", "V"=w598, "Vmax"=w583, "U"=w599, "Vmin"=w582) -> ("2D histogram or PDF"=w600:dbl[][], "U bin centre vals."=w580:dbl[], "V bin centre vals."=w579:dbl[], "UbinWidth"=w578:dbl, "VbinWidth"=w577:dbl)  [unwired: 1 out]
        "U bin centre vals." <- w580
        "V bin centre vals." <- w579
        "UbinWidth" <- w578
        "VbinWidth" <- w577
        n223 = case shown="2, Default" w605 {
          tunnel: [w616 w617] -> w603
          tunnel: w600 -> [w614 w617]
          frame 2, Default {
            n224 = local read "2D PDF"() -> (w615:dbl[][])
            n225 = Add(x=w615, y=w614) -> (x+y=w616:dbl[][])
          }
          frame 1 {
          }
        }
        "2D PDF" <- w603
        n226 = local write "U bin centre vals."(w580) -> ()
        n227 = local write "V bin centre vals."(w579) -> ()
        n228 = local write "UbinWidth"(w578) -> ()
        n229 = local write "VbinWidth"(w577) -> ()
      }
      frame "AutoCovariance" {
        n230 = Index Array(array=w625, index (row)=0) -> (element=w638:dbl[])  [unwired: 1 in]
        n231 = Index Array(array=w625, index (row)=1) -> (element=w632:dbl[])  [unwired: 1 in]
        n232 = Index Array(array=w625, index (row)=2) -> (element=w624:dbl[])  [unwired: 1 in]
        n233 = Index Array(array=w628, index (row)=0, index (col)=0 ("disabled index (col)")) -> (element=w636:dbl)
        n234 = Index Array(array=w628, index (row)=1, index (col)=0 ("disabled index (col)")) -> (element=w631:dbl)
        n235 = Index Array(array=w628, index (row)=2, index (col)=0 ("disabled index (col)")) -> (element=w623:dbl)
        n236 = Subtract(x=w624, y=w623) -> (x-y=w618:dbl[])
        n237 = Subtract(x=w638, y=w636) -> (x-y=w637:dbl[])
        n238 = Subtract(x=w632, y=w631) -> (x-y=w635:dbl[])
        n239 = call-poly <vilib>:"AutoCorrelation.vi"("normalization"=w620, "X"=w637) -> ("Rxx"=w639:dbl[])  [unwired: 9 out]
        n240 = call-poly <vilib>:"AutoCorrelation.vi"("normalization"=w620, "X"=w635) -> ("Rxx"=w634:dbl[])  [unwired: 9 out]
        n241 = call-poly <vilib>:"AutoCorrelation.vi"("normalization"=w620, "X"=w618) -> ("Rxx"=w621:dbl[])  [unwired: 9 out]
        n242 = case shown="2, Default" w619 {
          tunnel: [w660 w661] -> w642
          tunnel: w639 -> [w658 w661]
          frame 2, Default {
            n243 = local read "AutoCovariance of U"() -> (w659:dbl[])
            n244 = Add(x=w659, y=w658) -> (x+y=w660:dbl[])
          }
          frame 1 {
          }
        }
        "AutoCovariance of U" <- w642
        n245 = case shown="2, Default" w619 {
          tunnel: [w656 w657] -> w633
          tunnel: w634 -> [w654 w657]
          frame 2, Default {
            n246 = local read "AutoCovariance of V"() -> (w655:dbl[])
            n247 = Add(x=w655, y=w654) -> (x+y=w656:dbl[])
          }
          frame 1 {
          }
        }
        "AutoCovariance of V" <- w633
        n248 = case shown="2, Default" w619 {
          tunnel: [w652 w653] -> w622
          tunnel: w621 -> [w650 w653]
          frame 2, Default {
            n249 = local read "AutoCovariance of UV"() -> (w651:dbl[])
            n250 = Add(x=w651, y=w650) -> (x+y=w652:dbl[])
          }
          frame 1 {
          }
        }
        "AutoCovariance of UV" <- w622
      }
      frame "CrossCovariance" {
        n251 = Index Array(array=w676, index (row)=1) -> (element=w668:dbl[])  [unwired: 1 in]
        n252 = Index Array(array=w672, index (row)=0, index (col)=0 ("disabled index (col)")) -> (element=w670:dbl)
        n253 = Index Array(array=w676, index (row)=0) -> (element=w671:dbl[])  [unwired: 1 in]
        n254 = Index Array(array=w672, index (row)=1, index (col)=0 ("disabled index (col)")) -> (element=w667:dbl)
        n255 = Subtract(x=w671, y=w670) -> (x-y=w665:dbl[])
        n256 = Subtract(x=w668, y=w667) -> (x-y=w664:dbl[])
        n257 = call-poly <vilib>:"CrossCorrelation.vi"("normalization"=w663, "algorithm"=w662, "Y"=w664, "X"=w665) -> ("Rxy"=w666:dbl[])  [unwired: 7 out]
        n258 = case shown="2, Default" w669 {
          tunnel: [w687 w688] -> w675
          tunnel: w666 -> [w685 w688]
          frame 2, Default {
            n259 = local read "CrossCovariance"() -> (w686:dbl[])
            n260 = Add(x=w686, y=w685) -> (x+y=w687:dbl[])
          }
          frame 1 {
          }
        }
        "CrossCovariance" <- w675
      }
      frame "AutoPowerSpectrum" {
        n261 = Index Array(array=w697, index (row)=0) -> (element=w711:dbl[])  [unwired: 1 in]
        n262 = Index Array(array=w697, index (row)=1) -> (element=w708:dbl[])  [unwired: 1 in]
        n263 = Index Array(array=w697, index (row)=2) -> (element=w692:dbl[])  [unwired: 1 in]
        n264 = Index Array(array=w694, index (row)=0, index (col)=0 ("disabled index (col)")) -> (element=w710:dbl)
        n265 = Index Array(array=w694, index (row)=1, index (col)=0 ("disabled index (col)")) -> (element=w707:dbl)
        n266 = Index Array(array=w694, index (row)=2, index (col)=0 ("disabled index (col)")) -> (element=w693:dbl)
        n267 = Subtract(x=w711, y=w710) -> (x-y=w706:dbl[])
        n268 = Subtract(x=w708, y=w707) -> (x-y=w703:dbl[])
        n269 = Subtract(x=w692, y=w693) -> (x-y=w691:dbl[])
        n270 = call <vilib>:"Auto Power Spectrum.vi"("dt"=w690, "Signal (V)"=w706) -> ("df"=→"df APS":dbl, "Power Spectrum (V^2 rms)"=w704:dbl[])
        n271 = call <vilib>:"Auto Power Spectrum.vi"("dt"=w690, "Signal (V)"=w703) -> ("Power Spectrum (V^2 rms)"=w702:dbl[])  [unwired: 1 out]
        n272 = call <vilib>:"Auto Power Spectrum.vi"("dt"=w690, "Signal (V)"=w691) -> ("Power Spectrum (V^2 rms)"=w701:dbl[])  [unwired: 1 out]
        n273 = case shown="2, Default" w689 {
          tunnel: [w732 w733] -> w714
          tunnel: w704 -> [w730 w733]
          frame 2, Default {
            n274 = local read "PwrSpec of U"() -> (w731:dbl[])
            n275 = Add(x=w731, y=w730) -> (x+y=w732:dbl[])
          }
          frame 1 {
          }
        }
        "PwrSpec of U" <- w714
        n276 = case shown="2, Default" w689 {
          tunnel: [w728 w729] -> w709
          tunnel: w702 -> [w726 w729]
          frame 2, Default {
            n277 = local read "PwrSpec of V"() -> (w727:dbl[])
            n278 = Add(x=w727, y=w726) -> (x+y=w728:dbl[])
          }
          frame 1 {
          }
        }
        "PwrSpec of V" <- w709
        n279 = case shown="2, Default" w689 {
          tunnel: [w724 w725] -> w700
          tunnel: w701 -> [w722 w725]
          frame 2, Default {
            n280 = local read "PwrSpec of UV"() -> (w723:dbl[])
            n281 = Add(x=w723, y=w722) -> (x+y=w724:dbl[])
          }
          frame 1 {
          }
        }
        "PwrSpec of UV" <- w700
      }
      frame "CrossSpectrum" {
        n282 = Index Array(array=w750, index (row)=1) -> (element=w743:dbl[])  [unwired: 1 in]
        n283 = Index Array(array=w746, index (row)=0, index (col)=0 ("disabled index (col)")) -> (element=w744:dbl)
        n284 = Index Array(array=w750, index (row)=0) -> (element=w745:dbl[])  [unwired: 1 in]
        n285 = Index Array(array=w746, index (row)=1, index (col)=0 ("disabled index (col)")) -> (element=w742:dbl)
        n286 = Subtract(x=w745, y=w744) -> (x-y=w741:dbl[])
        n287 = Subtract(x=w743, y=w742) -> (x-y=w740:dbl[])
        n288 = call <vilib>:"Cross Power Spectrum.vi"("dt"=w739, "Signal Y (V)"=w740, "Signal X (V)"=w741) -> ("df"=→"df XPS":dbl, "Cross Power XY Spectrum Phase (radians)"=w735:dbl[], "Cross Power XY Spectrum Mag (V^2rms)"=w738:dbl[])
        n289 = case shown="2, Default" w736 {
          tunnel: [w765 w766] -> w749
          tunnel: w738 -> [w763 w766]
          frame 2, Default {
            n290 = local read "CrossPwrSpec"() -> (w764:dbl[])
            n291 = Add(x=w764, y=w763) -> (x+y=w765:dbl[])
          }
          frame 1 {
          }
        }
        "CrossPwrSpec" <- w749
        n292 = case shown="2, Default" w736 {
          tunnel: [w761 w762] -> w734
          tunnel: w735 -> [w760 w762]
          frame 2, Default {
            n293 = local read "CrossPhaseSpec"() -> (w759:dbl[])
            n294 = Add(x=w759, y=w760) -> (x+y=w761:dbl[])
          }
          frame 1 {
          }
        }
        "CrossPhaseSpec" <- w734
      }
      frame "D. Wavelet Xform (Morlet)" {
        n295 = Index Array(array=w782, index (row)=1) -> (element=w776:dbl[])  [unwired: 1 in]
        n296 = Index Array(array=w779, index (row)=0, index (col)=0 ("disabled index (col)")) -> (element=w777:dbl)
        n297 = Index Array(array=w782, index (row)=0) -> (element=w778:dbl[])  [unwired: 1 in]
        n298 = Index Array(array=w779, index (row)=1, index (col)=0 ("disabled index (col)")) -> (element=w775:dbl)
        n299 = Subtract(x=w778, y=w777) -> (x-y=w773:dbl[])
        n300 = Subtract(x=w776, y=w775) -> (x-y=w770:dbl[])
        n301 = call "DWT_morlet.vi"("dt"=w769, "1D Real input"=w773) -> ("Wavelet plot"=w772:dbl[][])  [unwired: 5 out]
        n302 = call "DWT_morlet.vi"("dt"=w769, "1D Real input"=w770) -> ("Wavelet plot"=w768:dbl[][])  [unwired: 5 out]
        n303 = case shown="2, Default" w774 {
          tunnel: [w797 w798] -> w771
          tunnel: w772 -> [w796 w798]
          frame 2, Default {
            n304 = local read "DWT U"() -> (w795:dbl[][])
            n305 = Add(x=w795, y=w796) -> (x+y=w797:dbl[][])
          }
          frame 1 {
          }
        }
        "DWT U" <- w771
        n306 = case shown="2, Default" w774 {
          tunnel: [w793 w794] -> w767
          tunnel: w768 -> [w792 w794]
          frame 2, Default {
            n307 = local read "DWT V"() -> (w791:dbl[][])
            n308 = Add(x=w791, y=w792) -> (x+y=w793:dbl[][])
          }
          frame 1 {
          }
        }
        "DWT V" <- w767
      }
      frame "Output" {
        w813 = string[] []
        n309 = for {
          tunnel: w818 -> [w834] mode=indexing
          tunnel: w817 -> [w833]
          shift-right: [w830] -> w815
          shift-left: w813 -> [w831]
          shift-right: [w828] -> w814
          shift-left: w813 -> [w829]
          tunnel: w807 -> [w827]
          tunnel: w806 -> [w826]
          tunnel: w805 -> [w825]
          tunnel: w804 -> [w824]
          tunnel: w803 -> [w823]
          tunnel: w802 -> [w822]
          tunnel: w801 -> [w821]
          tunnel: w800 -> [w820]
          tunnel: w799 -> [w819]
          n310 = Index Array(array=w833, index=w834) -> (element=w832:string)
          n311 = case shown="\"AutoCovariance\"" w832 {
            tunnel: w831 -> [w836 w850 w887 w941 w1031 w1050 w1332 w1400 w1470 w1486]
            tunnel: [w836 w849 w886 w941 w1031 w1049 w1332 w1400 w1470 w1486] -> w830
            tunnel: w829 -> [w835 w846 w885 w940 w1030 w1052 w1331 w1399 w1469 w1485]
            tunnel: [w835 w845 w884 w940 w1030 w1051 w1331 w1399 w1469 w1485] -> w828
            tunnel: w827 -> [_ w864 _ w937 w1026 w1058 w1328 w1396 w1466 _]
            tunnel: w826 -> [_ w854 _ w921 _ w1057 w1320 w1386 w1455 _]
            tunnel: w825 -> [_ _ _ _ _ w1055 w1314 w1369 w1443 _]
            tunnel: w824 -> [_ _ _ w908 _ _ _ _ _ _]
            tunnel: w823 -> [_ _ _ _ _ w1056 w1310 _ _ _]
            tunnel: w822 -> [_ w844 _ _ w1012 _ _ _ _ _]
            tunnel: w821 -> [_ _ _ _ w988 _ _ _ _ _]
            tunnel: w820 -> [_ w842 w882 _ w1008 w1054 _ _ _ _]
            tunnel: w819 -> [_ _ _ _ _ w1053 _ _ _ _]
            frame "False", Default {
            }
            frame "Moments to Order n" {
              n312 = global read "Meas_global.vi" "No of Analogue Samples"() -> (w853:i32)
              n313 = for {
                shift-right: [w871] -> w841
                shift-left: string[] [] -> [w870]
                tunnel: w844 -> [w872] mode=indexing
                tunnel: w842 -> [w869]
                n314 = Number To Fractional String(number=w872, precision (6)=w869) -> (F-format string=w873:string[])  [unwired: 2 out]
                n315 = Build Array (concatenate)(w870, w873) -> (w871:string[])
              }
              n316 = Multiply(x=w854, y=w853) -> (x*y=w855:i32)
              n317 = To Double Precision Float(number=w855) -> (double precision float=w856:dbl)
              n318 = local read "Moments"() -> (w848:dbl[])
              n319 = local read "2nd comp."() -> (w838:string)
              n320 = local read "format string"() -> (w860:string)
              n321 = Strip Path(path=w864) -> (name=w861:string)  [unwired: 1 out]
              n322 = Divide(x=w848, y=w856) -> (x/y=w839:dbl[])
              n323 = local read "Output Directory"() -> (w866:path)
              n324 = To Upper Case(1:w838) -> (0:w837:string)
              n325 = local write "Moments"(w839) -> ()
              n326 = case shown="\"V\", Default" w837 {
                tunnel: [string[] ["Mean:U:(m/s)", "Max:U:(m/s)", "Min:U:(m/s)", "Mean:W:(m/s)", "Max:W:(m/s)", "Min:W:(m/s)", "Mean:UW:(m/s)^2", "Max:UW:(m/s)^2", "Min:UW:(m/s)^2"] ("Plug in titles") string[] ["Mean:U:(m/s)", "Max:U:(m/s)", "Min:U:(m/s)", "Mean:V:(m/s)", "Max:V:(m/s)", "Min:V:(m/s)", "Mean:UV:(m/s)^2", "Max:UV:(m/s)^2", "Min:UV:(m/s)^2"] ("Plug in titles")] -> w840
                frame "W" {
                }
                frame "V", Default {
                }
              }
              n327 = Number To Fractional String(number=w839, precision (6)=w842) -> (F-format string=w847:string[])  [unwired: 2 out]
              n328 = Array To Spreadsheet String(array=w839, 3:w860) -> (spreadsheet string=w857:string)  [unwired: 1 out]
              n329 = local read "Moment labels"() -> (w852:string)
              n330 = while {
                shift-right: [w875] -> _
                shift-left: w852 -> [w878]
                tunnel: [w877] -> w851 mode=indexing
                stop <- w874 stop-if-true
                n331 = Search/Split String(string=w878, search string/char (-)="\t") -> (substring before match=w877:string, match + rest of string=w880:string)  [unwired: 2 out]
                n332 = call <vilib>:"Trim Whitespace.vi"("string"=w880) -> ("trimmed string"=w875:string)  [unwired: 1 in]
                n333 = String Length(string=w875) -> (length=w876:i32)
                n334 = Equal To 0?(x=w876) -> (x = 0?=w874:bool)
              }
              n335 = Concatenate Strings("Moms_" ("string"), w861) -> (w865:string)
              n336 = Build Path(base path=w866, name or relative path=w865) -> (appended path=w862:path)
              n337 = Format Into String(initial string=w852, "\r", w857) -> (resulting string=w859:string)  [unwired: 2 in, 1 out]
              n338 = Build Array (concatenate)(w850, w851, w840) -> (w849:string[])
              n339 = Build Array (concatenate)(w846, w847, w841) -> (w845:string[])
              n340 = Write to Text File(file (use dialog)=w862, text=w859) -> ()  [unwired: 1 in, 4 out]
            }
            frame "Quadrant Analysis" {
              n341 = local read "Quadrant probability"() -> (w883:dbl[])
              n342 = Number To Fractional String(number=w883, precision (6)=w882) -> (F-format string=w881:string[])  [unwired: 2 out]
              n343 = Build Array (concatenate)(w885, w881) -> (w884:string[])
              n344 = Build Array (concatenate)(w887, string[] ["Quadrant:Analysis:Q1", "Quadrant:Analysis:Q2", "Quadrant:Analysis:Q3", "Quadrant:Analysis:Q4"] ("Plug in titles")) -> (w886:string[])
            }
            frame "1D PDF" {
              n345 = local read "2nd comp."() -> (w892:string)
              n346 = To Upper Case(1:w892) -> (0:w891:string)
              n347 = local read "1D PDF UV"() -> (w920:dbl[])
              n348 = local read "1D PDF U"() -> (w922:dbl[])
              n349 = local read "1D PDF V"() -> (w923:dbl[])
              n350 = To Double Precision Float(number=w921) -> (double precision float=w914:dbl)
              n351 = local read "Axis UV"() -> (w917:dbl[])
              n352 = local read "Axis U"() -> (w932:dbl[])
              n353 = local read "Axis V"() -> (w929:dbl[])
              n354 = case shown="\"V\", Default" w891 {
                tunnel: ["pdfW_" ("string") "pdfV_" ("string")] -> w890
                tunnel: ["pdfUW_" ("string") "pdfUV_" ("string")] -> w889
                frame "W" {
                }
                frame "V", Default {
                }
              }
              n355 = case shown="True" w908 {
                tunnel: [w970 w974] -> w931
                tunnel: w922 -> [w970 w975]
                tunnel: w932 -> [_ w979]
                tunnel: w914 -> [_ w971]
                frame False {
                }
                frame True {
                  n356 = Index Array(array=w979, index=1) -> (element=w977:dbl)
                  n357 = Index Array(array=w979, index=0) -> (element=w976:dbl)
                  n358 = Subtract(x=w977, y=w976) -> (x-y=w973:dbl)
                  n359 = Multiply(x=w973, y=w971) -> (x*y=w972:dbl)
                  n360 = Divide(x=w975, y=w972) -> (x/y=w974:dbl[])
                }
              }
              n361 = case shown="True" w908 {
                tunnel: [w959 w963] -> w930
                tunnel: w923 -> [w959 w964]
                tunnel: w929 -> [_ w968]
                tunnel: w914 -> [_ w960]
                frame False {
                }
                frame True {
                  n362 = Index Array(array=w968, index=1) -> (element=w966:dbl)
                  n363 = Index Array(array=w968, index=0) -> (element=w965:dbl)
                  n364 = Subtract(x=w966, y=w965) -> (x-y=w962:dbl)
                  n365 = Multiply(x=w962, y=w960) -> (x*y=w961:dbl)
                  n366 = Divide(x=w964, y=w961) -> (x/y=w963:dbl[])
                }
              }
              n367 = case shown="True" w908 {
                tunnel: [w948 w952] -> w916
                tunnel: w920 -> [w948 w953]
                tunnel: w917 -> [_ w957]
                tunnel: w914 -> [_ w949]
                frame False {
                }
                frame True {
                  n368 = Index Array(array=w957, index=1) -> (element=w955:dbl)
                  n369 = Index Array(array=w957, index=0) -> (element=w954:dbl)
                  n370 = Subtract(x=w955, y=w954) -> (x-y=w951:dbl)
                  n371 = Multiply(x=w951, y=w949) -> (x*y=w950:dbl)
                  n372 = Divide(x=w953, y=w950) -> (x/y=w952:dbl[])
                }
              }
              n373 = Strip Path(path=w937) -> (name=w915:string)  [unwired: 1 out]
              n374 = local read "Output Directory"() -> (w939:path)
              n375 = local read "Output Directory"() -> (w926:path)
              n376 = local read "Output Directory"() -> (w913:path)
              n377 = Concatenate Strings("pdfU_" ("string"), w915) -> (w938:string)
              n378 = Concatenate Strings(w890, w915) -> (w924:string)
              n379 = Concatenate Strings(w889, w915) -> (w912:string)
              n380 = local read "format string"() -> (w893:string)
              n381 = Build Path(base path=w939, name or relative path=w938) -> (appended path=w935:path)
              n382 = Build Path(base path=w926, name or relative path=w924) -> (appended path=w925:path)
              n383 = Build Path(base path=w913, name or relative path=w912) -> (appended path=w911:path)
              n384 = Build Array(w932, w931) -> (w934:dbl[][])
              n385 = Build Array(w929, w930) -> (w927:dbl[][])
              n386 = Build Array(w917, w916) -> (w919:dbl[][])
              n387 = case shown="True" w908 {
                tunnel: ["hist." ("string") "pdf" ("string")] -> w894
                frame False {
                }
                frame True {
                }
              }
              n388 = Transpose 2D Array(2D array=w934) -> (transposed array=w933:dbl[][])
              n389 = Transpose 2D Array(2D array=w927) -> (transposed array=w928:dbl[][])
              n390 = Transpose 2D Array(2D array=w919) -> (transposed array=w918:dbl[][])
              n391 = Array To Spreadsheet String(array=w933, 3:w893) -> (spreadsheet string=w906:string)  [unwired: 1 out]
              n392 = Array To Spreadsheet String(array=w928, 3:w893) -> (spreadsheet string=w900:string)  [unwired: 1 out]
              n393 = Array To Spreadsheet String(array=w918, 3:w893) -> (spreadsheet string=w895:string)  [unwired: 1 out]
              n394 = Format Into String(initial string="binC" ("string"), "\t", w894, "\r", w900) -> (resulting string=w901:string)  [unwired: 2 in, 1 out]
              n395 = Format Into String(initial string="binC" ("string"), "\t", w894, "\r", w895) -> (resulting string=w896:string)  [unwired: 2 in, 1 out]
              n396 = Format Into String(initial string="binC" ("string"), "\t", w894, "\r", w906) -> (resulting string=w905:string)  [unwired: 2 in, 1 out]
              n397 = Write to Text File(file (use dialog)=w935, text=w905) -> ()  [unwired: 1 in, 4 out]
              n398 = Write to Text File(file (use dialog)=w925, text=w901) -> ()  [unwired: 1 in, 4 out]
              n399 = Write to Text File(file (use dialog)=w911, text=w896) -> ()  [unwired: 1 in, 4 out]
            }
            frame "2D PDF" {
              w1005 = "\r"
              # "Get XW cone line pts"
              # "N.B. wire 1 (single dot) gives +V, wire 2 (double dots) gives -V"
              n400 = local read "U bin centre vals."() -> (w1019:dbl[])
              n401 = local read "V bin centre vals."() -> (w1017:dbl[])
              n402 = local read "2nd comp."() -> (w983:string)
              n403 = local read "format string"() -> (w1011:string)
              n404 = Initialize Array(0.0 ("element"), 12 ("dimension size"), 2 ("dimension size")) -> (w992:dbl[][])
              n405 = Index Array(array=w1012, index (row)=0, index (col)=0 ("disabled index (col)")) -> (element=w985:dbl)
              n406 = Index Array(array=w1012, index (row)=1, index (col)=0 ("disabled index (col)")) -> (element=w987:dbl)
              n407 = Index Array(array=w1012, index (row)=0, index (col)=1 ("disabled index (col)")) -> (element=w990:dbl)
              n408 = local read "UbinWidth"() -> (w1010:dbl)
              n409 = local read "VbinWidth"() -> (w1018:dbl)
              n410 = local read "2D PDF"() -> (w1020:dbl[][])
              n411 = case shown="True" w988 {
                tunnel: w987 -> [_ w1037]
                tunnel: [0.0 w1036] -> w986
                tunnel: w985 -> [_ w1039]
                tunnel: [0.0 w1038] -> w984
                frame False {
                }
                frame True {
                  n412 = Negate(x=w1039) -> (-x=w1038:dbl)
                  n413 = Negate(x=w1037) -> (-x=w1036:dbl)
                }
              }
              n414 = To Upper Case(1:w983) -> (0:w982:string)
              n415 = case shown="\"V\", Default" w982 {
                tunnel: ["UbinW_WbinW_XWcone_2Ddata\n" ("initial string") "UbinW_VbinW_XWcone_2Ddata\n" ("initial string")] -> w981
                frame "W" {
                }
                frame "V", Default {
                }
              }
              n416 = for {
                tunnel: "Psi pull-out search strings" -> [w1041] mode=indexing
                tunnel: [w1040] -> w1003 mode=indexing
                n417 = global read "Dynamic_call_global.ph.vi" "Plug in values"() -> (w1042:string[])
                n418 = global read "Dynamic_call_global.ph.vi" "Plug in titles"() -> (w1044:string[])
                n419 = Match First String(2:w1044, 3:w1041) -> (0:w1043:i32)  [unwired: 1 out]
                n420 = Index String Array(1:w1043, 2:w1042) -> (0:w1040:string)  [unwired: 1 out]
              }
              n421 = Fract/Exp String To Number(string=w1003) -> (number=w996:dbl[])  [unwired: 4 out]
              n422 = expression code="Psi*pi/180.0"(w996) -> (w991:dbl[])
              n423 = formula code="float64 U1, mUmax, mU1 ;\nU1 = Umax + U0 ;\nmUmax = -Umax ;\nmU1 = mUmax + U0 ;\n//\n// Wire 1 mean cone\nPts[0][0] = mU1 ;   Pts[0][1] = (Umax / tan(Psis[0])) + V0 ;\nPts[1][0] = U1 ;      Pts[1][1] = (mUmax / tan(Psis[0])) + V0 ;\n// Wire 2 mean cone\nPts[2][0] = mU1 ;   Pts[2][1] = (mUmax / tan(Psis[1])) + V0 ;\nPts[3][0] = U1 ;      Pts[3][1] = (Umax / tan(Psis[1])) + V0 ;\n// Wire 1 max cone\nPts[4][0] = mU1 ;   Pts[4][1] = (Umax / tan(Psis[2])) + V0 ;\nPts[5][0] = U1 ;      Pts[5][1] = (mUmax / tan(Psis[2])) + V0 ;\n// Wire 1 min cone\nPts[6][0] = mU1 ;   Pts[6][1] = (Umax / tan(Psis[3])) + V0 ;\nPts[7][0] = U1 ;      Pts[7][1] = (mUmax / tan(Psis[3])) + V0 ;\n// Wire 2 max cone\nPts[8][0] = mU1 ;   Pts[8][1] = (mUmax / tan(Psis[4])) + V0 ;\nPts[9][0] = U1 ;      Pts[9][1] = (Umax / tan(Psis[4])) + V0 ;\n// Wire 2 min cone\nPts[10][0] = mU1 ; Pts[10][1] = (mUmax / tan(Psis[5])) + V0 ;\nPts[11][0] = U1 ;    Pts[11][1] = (Umax / tan(Psis[5])) + V0 ;"("Pts"=w992, "U0"=w984, "V0"=w986, "Umax"=w990, "Psis"=w991) -> ("Pts"=w989:dbl[][])
              n424 = Number To Fractional String(number=w1010, precision (6)=w1008) -> (F-format string=w1009:string)  [unwired: 2 out]
              n425 = Number To Fractional String(number=w1018, precision (6)=w1008) -> (F-format string=w1015:string)  [unwired: 2 out]
              n426 = for {
                tunnel: w1020 -> [w1045] mode=indexing
                tunnel: w1019 -> [w1047] mode=indexing
                tunnel: [w1046] -> w1016 mode=indexing
                n427 = Insert Into Array(array=w1045, index=0, new element=w1047) -> (w1046:dbl[])
              }
              n428 = Array To Spreadsheet String(array=w1017, 3:w1011) -> (spreadsheet string=w1023:string)  [unwired: 1 out]
              n429 = Format Into String(initial string="\t", w1023) -> (resulting string=w1013:string)  [unwired: 2 in, 1 out]
              n430 = Strip Path(path=w1026) -> (name=w1028:string)  [unwired: 1 out]
              n431 = local read "Output Directory"() -> (w1029:path)
              n432 = Array To Spreadsheet String(array=w1016, 3:w1011) -> (spreadsheet string=w1014:string)  [unwired: 1 out]
              n433 = Concatenate Strings("2DPDF_" ("string"), w1028) -> (w1027:string)
              n434 = Build Path(base path=w1029, name or relative path=w1027) -> (appended path=w1021:path)
              n435 = Array To Spreadsheet String(array=w989, 3:w1011) -> (spreadsheet string=w1006:string)  [unwired: 1 out]
              n436 = Format Into String(initial string=w981, w1005, w1009, w1005, w1015, w1005, w1005, w1006, w1005) -> (resulting string=w1007:string)  [unwired: 2 in, 1 out]
              n437 = Concatenate Strings(w1007, w1013, w1014) -> (w1022:string)
              n438 = Write to Text File(file (use dialog)=w1021, text=w1022) -> ()  [unwired: 1 in, 4 out]
            }
            frame "AutoCovariance" {
              n439 = stacked-sequence {
                seq-local: [w1077 _ _] -> [_ w1156 _]
                seq-local: [w1076 _ _] -> [_ w1155 _]
                seq-local: [w1075 _ _] -> [_ w1154 _]
                seq-local: [w1069 _ _] -> [_ w1146 _]
                seq-local: [w1066 _ _] -> [_ w1139 _]
                seq-local: [w1065 _ _] -> [_ w1133 _]
                seq-local: [w1074 _ _] -> [_ w1162 _]
                seq-local: [w1073 _ _] -> [_ w1169 _]
                seq-local: [w1072 _ _] -> [_ w1165 _]
                seq-local: [w1071 _ _] -> [_ w1163 _]
                seq-local: [_ w1129 _] -> [_ _ w1271]
                seq-local: [_ w1128 _] -> [_ _ w1270]
                seq-local: [_ w1127 _] -> [_ _ w1269]
                seq-local: [_ w1126 _] -> [_ _ w1296]
                seq-local: [_ w1125 _] -> [_ _ w1295]
                seq-local: [_ w1124 _] -> [_ _ w1293]
                tunnel: w1058 -> [w1101 _ _]
                tunnel: w1057 -> [w1093 _ w1299]
                tunnel: w1056 -> [w1086 w1157 w1292]
                tunnel: w1055 -> [w1078 w1167 _]
                tunnel: w1054 -> [_ w1147 w1278]
                tunnel: w1053 -> [_ _ w1255]
                tunnel: w1052 -> [_ _ w1223]
                tunnel: [_ _ w1267] -> w1051
                tunnel: w1050 -> [_ _ w1266]
                tunnel: [_ _ w1265] -> w1049
                frame #0 {
                  # "This frame gets the Acov arrays"
                  n440 = To Double Precision Float(number=w1093) -> (double precision float=w1079:dbl)
                  n441 = local read "AutoCovariance of U"() -> (w1092:dbl[])
                  n442 = local read "AutoCovariance of UV"() -> (w1063:dbl[])
                  n443 = local read "AutoCovariance of V"() -> (w1089:dbl[])
                  n444 = local read "2nd comp."() -> (w1062:string)
                  n445 = local read "format string"() -> (w1064:string)
                  n446 = To Upper Case(1:w1062) -> (0:w1061:string)
                  n447 = Strip Path(path=w1101) -> (name=w1080:string)  [unwired: 1 out]
                  n448 = case shown="\"V\", Default" w1061 {
                    tunnel: ["AcovW_" ("string") "AcovV_" ("string")] -> w1060
                    tunnel: ["AcovUW_" ("string") "AcovUV_" ("string")] -> w1059
                    frame "W" {
                    }
                    frame "V", Default {
                    }
                  }
                  n449 = local read "Output Directory"() -> (w1095:path)
                  n450 = local read "Output Directory"() -> (w1083:path)
                  n451 = Array Size(array=w1092) -> (size(s)=w1088:i32)
                  n452 = expression code="(N-1)/2"(w1088) -> (w1074:i32)
                  n453 = case shown="True" w1078 {
                    tunnel: w1089 -> [_ w1115]
                    tunnel: w1074 -> [_ w1114]
                    tunnel: w1079 -> [w1112 _]
                    tunnel: [w1112 w1113] -> w1090
                    frame False {
                    }
                    frame True {
                      n454 = Index Array(array=w1115, index=w1114) -> (element=w1113:dbl)
                    }
                  }
                  n455 = case shown="True" w1078 {
                    tunnel: w1063 -> [_ w1111]
                    tunnel: w1074 -> [_ w1110]
                    tunnel: w1079 -> [w1108 _]
                    tunnel: [w1108 w1109] -> w1085
                    frame False {
                    }
                    frame True {
                      n456 = Index Array(array=w1111, index=w1110) -> (element=w1109:dbl)
                    }
                  }
                  n457 = case shown="True" w1078 {
                    tunnel: w1092 -> [_ w1119]
                    tunnel: w1074 -> [_ w1118]
                    tunnel: w1079 -> [w1116 _]
                    tunnel: [w1116 w1117] -> w1091
                    frame False {
                    }
                    frame True {
                      n458 = Index Array(array=w1119, index=w1118) -> (element=w1117:dbl)
                    }
                  }
                  n459 = Divide(x=w1089, y=w1090) -> (x/y=w1072:dbl[])
                  n460 = Divide(x=w1063, y=w1085) -> (x/y=w1071:dbl[])
                  n461 = Divide(x=w1092, y=w1091) -> (x/y=w1073:dbl[])
                  n462 = local read "Output Directory"() -> (w1103:path)
                  n463 = Negate(x=w1074) -> (-x=w1087:i32)
                  n464 = Concatenate Strings(w1060, w1080) -> (w1096:string)
                  n465 = To Double Precision Float(number=w1087) -> (double precision float=w1098:dbl)
                  n466 = Concatenate Strings(w1059, w1080) -> (w1082:string)
                  n467 = Multiply(x=w1098, y=w1086) -> (x*y=w1099:dbl)
                  n468 = Build Path(base path=w1095, name or relative path=w1096) -> (appended path=w1076:path)
                  n469 = Build Path(base path=w1083, name or relative path=w1082) -> (appended path=w1075:path)
                  n470 = Concatenate Strings("AcovU_" ("string"), w1080) -> (w1102:string)
                  n471 = for {
                    N: w1088 -> [_]
                    shift-right: [w1122] -> _
                    shift-left: w1099 -> [w1120]
                    tunnel: w1086 -> [w1121]
                    tunnel: [w1120] -> w1081 mode=indexing
                    n472 = Add(x=w1120, y=w1121) -> (x+y=w1122:dbl)
                  }
                  n473 = Build Array(w1081, w1073) -> (w1097:dbl[][])
                  n474 = Build Array(w1081, w1072) -> (w1094:dbl[][])
                  n475 = Build Array(w1081, w1071) -> (w1084:dbl[][])
                  n476 = Transpose 2D Array(2D array=w1097) -> (transposed array=w1070:dbl[][])
                  n477 = Transpose 2D Array(2D array=w1094) -> (transposed array=w1068:dbl[][])
                  n478 = Transpose 2D Array(2D array=w1084) -> (transposed array=w1067:dbl[][])
                  n479 = Array To Spreadsheet String(array=w1070, 3:w1064) -> (spreadsheet string=w1069:string)  [unwired: 1 out]
                  n480 = Array To Spreadsheet String(array=w1068, 3:w1064) -> (spreadsheet string=w1066:string)  [unwired: 1 out]
                  n481 = Array To Spreadsheet String(array=w1067, 3:w1064) -> (spreadsheet string=w1065:string)  [unwired: 1 out]
                  n482 = Build Path(base path=w1103, name or relative path=w1102) -> (appended path=w1077:path)
                }
                frame #1 {
                  w1135 = "\r"
                  w1144 = "\r"
                  w1149 = "\r"
                  w1159 = 0.0
                  # "block integrate to zero-crossing"
                  # "This frame gets the tscales"
                  # "midIndex"
                  # "AcovUV"
                  # "AcovV"
                  # "AcovU"
                  n483 = Array Subset(array=w1165, index=w1162) -> (w1164:dbl[])  [unwired: 1 in]
                  n484 = Array Subset(array=w1163, index=w1162) -> (w1161:dbl[])  [unwired: 1 in]
                  n485 = Array Subset(array=w1169, index=w1162) -> (w1168:dbl[])  [unwired: 1 in]
                  n486 = case shown="False" w1167 {
                    tunnel: w1168 -> [w1202 w1206]
                    tunnel: [w1200 w1206] -> w1166
                    tunnel: w1164 -> [w1197 w1205]
                    tunnel: w1161 -> [w1193 w1204]
                    tunnel: [w1196 w1205] -> w1158
                    tunnel: [w1192 w1204] -> w1160
                    frame False {
                      n487 = Index Array(array=w1202, index=0) -> (element=w1201:dbl)
                      n488 = Index Array(array=w1197, index=0) -> (element=w1199:dbl)
                      n489 = Index Array(array=w1193, index=0) -> (element=w1195:dbl)
                      n490 = Divide(x=w1202, y=w1201) -> (x/y=w1200:dbl[])
                      n491 = Divide(x=w1197, y=w1199) -> (x/y=w1196:dbl[])
                      n492 = Divide(x=w1193, y=w1195) -> (x/y=w1192:dbl[])
                    }
                    frame True {
                    }
                  }
                  n493 = while {
                    tunnel: w1166 -> [w1211] mode=indexing
                    shift-right: [w1210] -> w1148
                    shift-left: w1159 -> [w1208]
                    stop <- w1209 continue-if-true
                    n494 = Greater Than 0?(x=w1211) -> (x > 0?=w1207:bool)
                    n495 = case shown="True" w1207 {
                      tunnel: w1211 -> [_ w1217]
                      tunnel: [w1212 w1216] -> w1210
                      tunnel: [FALSE TRUE] -> w1209
                      tunnel: w1208 -> [w1212 w1214]
                      frame False {
                      }
                      frame True {
                        n496 = Add(x=w1217, y=w1214) -> (x+y=w1216:dbl)
                      }
                    }
                  }
                  n497 = while {
                    tunnel: w1158 -> [w1185] mode=indexing
                    shift-right: [w1184] -> w1130
                    shift-left: w1159 -> [w1182]
                    stop <- w1183 continue-if-true
                    n498 = Greater Than 0?(x=w1185) -> (x > 0?=w1181:bool)
                    n499 = case shown="True" w1181 {
                      tunnel: w1185 -> [_ w1191]
                      tunnel: [w1186 w1190] -> w1184
                      tunnel: [FALSE TRUE] -> w1183
                      tunnel: w1182 -> [w1186 w1188]
                      frame False {
                      }
                      frame True {
                        n500 = Add(x=w1191, y=w1188) -> (x+y=w1190:dbl)
                      }
                    }
                  }
                  n501 = while {
                    tunnel: w1160 -> [w1174] mode=indexing
                    shift-right: [w1173] -> w1123
                    shift-left: w1159 -> [w1171]
                    stop <- w1172 continue-if-true
                    n502 = Greater Than 0?(x=w1174) -> (x > 0?=w1170:bool)
                    n503 = case shown="True" w1170 {
                      tunnel: w1174 -> [_ w1180]
                      tunnel: [w1175 w1179] -> w1173
                      tunnel: [FALSE TRUE] -> w1172
                      tunnel: w1171 -> [w1175 w1177]
                      frame False {
                      }
                      frame True {
                        n504 = Add(x=w1180, y=w1177) -> (x+y=w1179:dbl)
                      }
                    }
                  }
                  n505 = Multiply(x=w1130, y=w1157) -> (x*y=w1125:dbl)
                  n506 = Multiply(x=w1123, y=w1157) -> (x*y=w1124:dbl)
                  n507 = Multiply(x=w1148, y=w1157) -> (x*y=w1126:dbl)
                  n508 = Number To Fractional String(number=w1126, precision (6)=w1147) -> (F-format string=w1129:string)  [unwired: 2 out]
                  n509 = Format Into String(initial string="avg. tscale(s)" ("string"), w1149, w1129, w1149, w1149, "t_lag(s)" ("string"), "\t", "Acov." ("string"), w1149, w1146) -> (resulting string=w1145:string)  [unwired: 2 in, 1 out]
                  n510 = Number To Fractional String(number=w1125, precision (6)=w1147) -> (F-format string=w1128:string)  [unwired: 2 out]
                  n511 = Format Into String(initial string="avg. tscale(s)" ("string"), w1144, w1128, w1144, w1144, "t_lag(s)" ("string"), "\t", "Acov." ("string"), w1144, w1139) -> (resulting string=w1132:string)  [unwired: 2 in, 1 out]
                  n512 = Number To Fractional String(number=w1124, precision (6)=w1147) -> (F-format string=w1127:string)  [unwired: 2 out]
                  n513 = Format Into String(initial string="avg. tscale(s)" ("string"), w1135, w1127, w1135, w1135, "t_lag(s)" ("string"), "\t", "Acov." ("string"), w1135, w1133) -> (resulting string=w1131:string)  [unwired: 2 in, 1 out]
                  n514 = Write to Text File(file (use dialog)=w1156, text=w1145) -> ()  [unwired: 1 in, 4 out]
                  n515 = Write to Text File(file (use dialog)=w1155, text=w1132) -> ()  [unwired: 1 in, 4 out]
                  n516 = Write to Text File(file (use dialog)=w1154, text=w1131) -> ()  [unwired: 1 in, 4 out]
                }
                frame #2 {
                  # "std err in var"
                  # "wire order:\nU\nV\nUV"
                  # "std err in mean"
                  # "N independent samples"
                  # "tcU\ntcV\ntcUV"
                  n517 = global read "Meas_global.vi" "No of Analogue Samples"() -> (w1298:i32)
                  n518 = local read "Moments"() -> (w1252:dbl[])
                  n519 = Reciprocal(x=w1292) -> (1/x=w1294:dbl)
                  n520 = Decrement(x=w1255) -> (x-1=w1258:i32)
                  n521 = Multiply(x=w1296, y=w1294) -> (x*y=w1291:dbl)
                  n522 = Multiply(x=w1295, y=w1294) -> (x*y=w1289:dbl)
                  n523 = Multiply(x=w1293, y=w1294) -> (x*y=w1290:dbl)
                  n524 = Add(x=w1258, y=w1258) -> (x+y=w1259:i32)
                  n525 = Multiply(x=w1299, y=w1298) -> (x*y=w1297:i32)
                  n526 = Index Array(array=w1252, index=0) -> (element=w1251:dbl)
                  n527 = Index Array(array=w1252, index=w1258) -> (element=w1250:dbl)
                  n528 = Index Array(array=w1252, index=w1259) -> (element=w1249:dbl)
                  n529 = To Double Precision Float(number=w1297) -> (double precision float=w1288:dbl)
                  n530 = Subtract(x=w1288, y=w1291) -> (x-y=w1287:dbl)
                  n531 = Subtract(x=w1288, y=w1289) -> (x-y=w1286:dbl)
                  n532 = Subtract(x=w1288, y=w1290) -> (x-y=w1285:dbl)
                  n533 = Round Toward -Infinity(1:w1287) -> (0:w1235:dbl)
                  n534 = Divide(x=w1251, y=w1235) -> (x/y=w1283:dbl)
                  n535 = Square Root(x=w1283) -> (sqrt(x)=w1281:dbl)
                  n536 = Round Toward -Infinity(1:w1286) -> (0:w1222:dbl)
                  n537 = Divide(x=w1250, y=w1222) -> (x/y=w1282:dbl)
                  n538 = Square Root(x=w1282) -> (sqrt(x)=w1280:dbl)
                  n539 = Round Toward -Infinity(1:w1285) -> (0:w1219:dbl)
                  n540 = Divide(x=w1249, y=w1219) -> (x/y=w1264:dbl)
                  n541 = Absolute Value(x=w1264) -> (abs(x)=w1263:dbl)
                  n542 = Square Root(x=w1263) -> (sqrt(x)=w1279:dbl)
                  n543 = Add(x=w1259, y=w1258) -> (x+y=w1257:i32)
                  n544 = local read "2nd comp."() -> (w1262:string)
                  n545 = Increment(x=w1255) -> (x+1=w1254:i32)
                  n546 = Increment(x=w1257) -> (x+1=w1256:i32)
                  n547 = expression code="N0-3"(w1235) -> (w1247:dbl)
                  n548 = expression code="N0-1"(w1235) -> (w1246:dbl)
                  n549 = expression code="N0-3"(w1222) -> (w1244:dbl)
                  n550 = expression code="N0-1"(w1222) -> (w1245:dbl)
                  n551 = expression code="N0-3"(w1219) -> (w1243:dbl)
                  n552 = expression code="N0-1"(w1219) -> (w1242:dbl)
                  n553 = Square(x=w1251) -> (x^2=w1240:dbl)
                  n554 = Square(x=w1250) -> (x^2=w1234:dbl)
                  n555 = Square(x=w1249) -> (x^2=w1230:dbl)
                  n556 = Divide(x=w1247, y=w1246) -> (x/y=w1239:dbl)
                  n557 = Divide(x=w1244, y=w1245) -> (x/y=w1233:dbl)
                  n558 = Divide(x=w1243, y=w1242) -> (x/y=w1229:dbl)
                  n559 = Index Array(array=w1252, index=2) -> (element=w1248:dbl)
                  n560 = Index Array(array=w1252, index=w1254) -> (element=w1232:dbl)
                  n561 = Index Array(array=w1252, index=w1256) -> (element=w1227:dbl)
                  n562 = To Upper Case(1:w1262) -> (0:w1261:string)
                  n563 = Multiply(x=w1240, y=w1239) -> (x*y=w1241:dbl)
                  n564 = Multiply(x=w1234, y=w1233) -> (x*y=w1231:dbl)
                  n565 = Multiply(x=w1230, y=w1229) -> (x*y=w1228:dbl)
                  n566 = case shown="\"V\", Default" w1261 {
                    tunnel: [string[] ["Std. err.:U:(m/s)", "Std. err.:W:(m/s)", "Std. err.:UW:(m/s)", "Std. err.:u^2:(m/s)^2", "Std. err.:w^2:(m/s)^2", "Std. err.:uw:(m/s)^2", "Integ. tscale:U:(s)", "Integ. tscale:W:(s)", "Integ. tscale:UW:(s)"] ("Plug in titles") string[] ["Std. err.:U:(m/s)", "Std. err.:V:(m/s)", "Std. err.:UV:(m/s)", "Std. err.:u^2:(m/s)^2", "Std. err.:v^2:(m/s)^2", "Std. err.:uv:(m/s)^2", "Integ. tscale:U:(s)", "Integ. tscale:V:(s)", "Integ. tscale:UV:(s)"] ("Plug in titles")] -> w1260
                    frame "W" {
                    }
                    frame "V", Default {
                    }
                  }
                  n567 = Subtract(x=w1248, y=w1241) -> (x-y=w1238:dbl)
                  n568 = Subtract(x=w1232, y=w1231) -> (x-y=w1226:dbl)
                  n569 = Subtract(x=w1227, y=w1228) -> (x-y=w1220:dbl)
                  n570 = Number To Fractional String(number=w1281, precision (6)=w1278) -> (F-format string=w1277:string)  [unwired: 2 out]
                  n571 = Number To Fractional String(number=w1280, precision (6)=w1278) -> (F-format string=w1276:string)  [unwired: 2 out]
                  n572 = Number To Fractional String(number=w1279, precision (6)=w1278) -> (F-format string=w1275:string)  [unwired: 2 out]
                  n573 = Divide(x=w1238, y=w1235) -> (x/y=w1237:dbl)
                  n574 = Divide(x=w1226, y=w1222) -> (x/y=w1225:dbl)
                  n575 = Divide(x=w1220, y=w1219) -> (x/y=w1221:dbl)
                  n576 = Square Root(x=w1237) -> (sqrt(x)=w1236:dbl)
                  n577 = Square Root(x=w1225) -> (sqrt(x)=w1224:dbl)
                  n578 = Square Root(x=w1221) -> (sqrt(x)=w1218:dbl)
                  n579 = Number To Fractional String(number=w1236, precision (6)=w1278) -> (F-format string=w1274:string)  [unwired: 2 out]
                  n580 = Number To Fractional String(number=w1224, precision (6)=w1278) -> (F-format string=w1273:string)  [unwired: 2 out]
                  n581 = Number To Fractional String(number=w1218, precision (6)=w1278) -> (F-format string=w1272:string)  [unwired: 2 out]
                  n582 = Build Array(w1277, w1276, w1275, w1274, w1273, w1272, w1271, w1270, w1269) -> (w1268:string[])
                  n583 = Build Array (concatenate)(w1268, w1223) -> (w1267:string[])
                  n584 = Build Array (concatenate)(w1260, w1266) -> (w1265:string[])
                }
              }
            }
            frame "CrossCovariance" {
              n585 = To Double Precision Float(number=w1320) -> (double precision float=w1315:dbl)
              n586 = local read "CrossCovariance"() -> (w1317:dbl[])
              n587 = local read "format string"() -> (w1321:string)
              n588 = local read "2nd comp."() -> (w1304:string)
              n589 = To Upper Case(1:w1304) -> (0:w1303:string)
              n590 = Strip Path(path=w1328) -> (name=w1322:string)  [unwired: 1 out]
              n591 = case shown="\"V\", Default" w1303 {
                tunnel: ["XcovUW_" ("string") "XcovUV_" ("string")] -> w1302
                frame "W" {
                }
                frame "V", Default {
                }
              }
              n592 = Array Size(array=w1317) -> (size(s)=w1313:i32)
              n593 = expression code="(N-1)/2"(w1313) -> (w1312:i32)
              n594 = case shown="True" w1314 {
                tunnel: w1317 -> [_ w1338]
                tunnel: w1312 -> [_ w1337]
                tunnel: w1315 -> [w1335 _]
                tunnel: [w1335 w1336] -> w1316
                frame False {
                }
                frame True {
                  n595 = Index Array(array=w1338, index=w1337) -> (element=w1336:dbl)
                }
              }
              n596 = Divide(x=w1317, y=w1316) -> (x/y=w1319:dbl[])
              n597 = local read "Output Directory"() -> (w1330:path)
              n598 = Negate(x=w1312) -> (-x=w1311:i32)
              n599 = To Double Precision Float(number=w1311) -> (double precision float=w1325:dbl)
              n600 = Multiply(x=w1325, y=w1310) -> (x*y=w1326:dbl)
              n601 = Concatenate Strings(w1302, w1322) -> (w1329:string)
              n602 = for {
                N: w1313 -> [_]
                shift-right: [w1341] -> _
                shift-left: w1326 -> [w1339]
                tunnel: w1310 -> [w1340]
                tunnel: [w1339] -> w1318 mode=indexing
                n603 = Add(x=w1339, y=w1340) -> (x+y=w1341:dbl)
              }
              n604 = Build Array(w1318, w1319) -> (w1324:dbl[][])
              n605 = Transpose 2D Array(2D array=w1324) -> (transposed array=w1323:dbl[][])
              n606 = Array To Spreadsheet String(array=w1323, 3:w1321) -> (spreadsheet string=w1306:string)  [unwired: 1 out]
              n607 = Build Path(base path=w1330, name or relative path=w1329) -> (appended path=w1327:path)
              n608 = Format Into String(initial string="t_lag(s)" ("string"), "\t", w1302, "\r", w1306) -> (resulting string=w1305:string)  [unwired: 2 in, 1 out]
              n609 = Write to Text File(file (use dialog)=w1327, text=w1305) -> ()  [unwired: 1 in, 4 out]
            }
            frame "AutoPowerSpectrum" {
              n610 = To Double Precision Float(number=w1386) -> (double precision float=w1364:dbl)
              n611 = local read "PwrSpec of U"() -> (w1380:dbl[])
              n612 = local read "2nd comp."() -> (w1347:string)
              n613 = local read "format string"() -> (w1368:string)
              n614 = local read "PwrSpec of UV"() -> (w1377:dbl[])
              n615 = local read "PwrSpec of V"() -> (w1378:dbl[])
              n616 = To Upper Case(1:w1347) -> (0:w1346:string)
              n617 = Strip Path(path=w1396) -> (name=w1366:string)  [unwired: 1 out]
              n618 = case shown="\"V\", Default" w1346 {
                tunnel: ["PwrSpecW_" ("string") "PwrSpecV_" ("string")] -> w1345
                tunnel: ["PwrSpecUW_" ("string") "PwrSpecUV_" ("string")] -> w1343
                tunnel: ["non-dim w^2" ("string") "non-dim v^2" ("string")] -> w1344
                tunnel: ["non-dim (uw)^2" ("string") "non-dim (uv)^2" ("string")] -> w1342
                frame "W" {
                }
                frame "V", Default {
                }
              }
              n619 = local read "df APS"() -> (w1365:dbl)
              n620 = case shown="True" w1369 {
                tunnel: w1364 -> [w1419 _]
                tunnel: [w1419 w1421] -> w1381
                tunnel: w1365 -> [_ w1422]
                tunnel: w1380 -> [_ w1420]
                frame False {
                }
                frame True {
                  n621 = Add Array Elements(numeric array=w1420) -> (sum=w1423:dbl)
                  n622 = Multiply(x=w1423, y=w1422) -> (x*y=w1421:dbl)
                }
              }
              n623 = case shown="True" w1369 {
                tunnel: w1364 -> [w1414 _]
                tunnel: [w1414 w1416] -> w1379
                tunnel: w1365 -> [_ w1417]
                tunnel: w1378 -> [_ w1415]
                frame False {
                }
                frame True {
                  n624 = Add Array Elements(numeric array=w1415) -> (sum=w1418:dbl)
                  n625 = Multiply(x=w1418, y=w1417) -> (x*y=w1416:dbl)
                }
              }
              n626 = case shown="True" w1369 {
                tunnel: w1364 -> [w1409 _]
                tunnel: [w1409 w1411] -> w1376
                tunnel: w1365 -> [_ w1412]
                tunnel: w1377 -> [_ w1410]
                frame False {
                }
                frame True {
                  n627 = Add Array Elements(numeric array=w1410) -> (sum=w1413:dbl)
                  n628 = Multiply(x=w1413, y=w1412) -> (x*y=w1411:dbl)
                }
              }
              n629 = Divide(x=w1380, y=w1381) -> (x/y=w1385:dbl[])
              n630 = Divide(x=w1378, y=w1379) -> (x/y=w1384:dbl[])
              n631 = Divide(x=w1377, y=w1376) -> (x/y=w1375:dbl[])
              n632 = Array Size(array=w1380) -> (size(s)=w1383:i32)
              n633 = local read "Output Directory"() -> (w1398:path)
              n634 = local read "Output Directory"() -> (w1390:path)
              n635 = local read "Output Directory"() -> (w1371:path)
              n636 = expression code="0.5*df"(w1365) -> (w1382:dbl)
              n637 = Concatenate Strings("PwrSpecU_" ("string"), w1366) -> (w1397:string)
              n638 = Concatenate Strings(w1345, w1366) -> (w1391:string)
              n639 = Concatenate Strings(w1343, w1366) -> (w1370:string)
              n640 = for {
                N: w1383 -> [_]
                shift-right: [w1426] -> _
                shift-left: w1382 -> [w1424]
                tunnel: w1365 -> [w1425]
                tunnel: [w1424] -> w1367 mode=indexing
                n641 = Add(x=w1424, y=w1425) -> (x+y=w1426:dbl)
              }
              n642 = Build Array(w1367, w1385) -> (w1393:dbl[][])
              n643 = Build Array(w1367, w1384) -> (w1387:dbl[][])
              n644 = Build Array(w1367, w1375) -> (w1374:dbl[][])
              n645 = Transpose 2D Array(2D array=w1393) -> (transposed array=w1392:dbl[][])
              n646 = Transpose 2D Array(2D array=w1387) -> (transposed array=w1388:dbl[][])
              n647 = Transpose 2D Array(2D array=w1374) -> (transposed array=w1373:dbl[][])
              n648 = Array To Spreadsheet String(array=w1392, 3:w1368) -> (spreadsheet string=w1359:string)  [unwired: 1 out]
              n649 = Array To Spreadsheet String(array=w1388, 3:w1368) -> (spreadsheet string=w1351:string)  [unwired: 1 out]
              n650 = Array To Spreadsheet String(array=w1373, 3:w1368) -> (spreadsheet string=w1350:string)  [unwired: 1 out]
              n651 = Build Path(base path=w1398, name or relative path=w1397) -> (appended path=w1394:path)
              n652 = Build Path(base path=w1390, name or relative path=w1391) -> (appended path=w1389:path)
              n653 = Build Path(base path=w1371, name or relative path=w1370) -> (appended path=w1372:path)
              n654 = Format Into String(initial string="f (Hz)" ("string"), "\t", w1342, "\r", w1350) -> (resulting string=w1349:string)  [unwired: 2 in, 1 out]
              n655 = Format Into String(initial string="f (Hz)" ("string"), "\t", "non-dim u^2" ("string"), "\r", w1359) -> (resulting string=w1358:string)  [unwired: 2 in, 1 out]
              n656 = Format Into String(initial string="f (Hz)" ("string"), "\t", w1344, "\r", w1351) -> (resulting string=w1348:string)  [unwired: 2 in, 1 out]
              n657 = Write to Text File(file (use dialog)=w1394, text=w1358) -> ()  [unwired: 1 in, 4 out]
              n658 = Write to Text File(file (use dialog)=w1389, text=w1348) -> ()  [unwired: 1 in, 4 out]
              n659 = Write to Text File(file (use dialog)=w1372, text=w1349) -> ()  [unwired: 1 in, 4 out]
            }
            frame "CrossSpectrum" {
              n660 = To Double Precision Float(number=w1455) -> (double precision float=w1445:dbl)
              n661 = local read "CrossPwrSpec"() -> (w1447:dbl[])
              n662 = local read "CrossPhaseSpec"() -> (w1449:dbl[])
              n663 = local read "2nd comp."() -> (w1431:string)
              n664 = local read "format string"() -> (w1456:string)
              n665 = expression code="X*180.0/pi"(w1449) -> (w1448:dbl[])
              n666 = To Upper Case(1:w1431) -> (0:w1430:string)
              n667 = Strip Path(path=w1466) -> (name=w1459:string)  [unwired: 1 out]
              n668 = case shown="\"V\", Default" w1430 {
                tunnel: ["XPwrSpecUW_" ("string") "XPwrSpecUV_" ("string")] -> w1429
                tunnel: ["XPhiSpecUW_" ("string") "XPhiSpecUV_" ("string")] -> w1427
                tunnel: ["non-dim u^2w^2." ("string") "non-dim u^2v^2." ("string")] -> w1428
                frame "W" {
                }
                frame "V", Default {
                }
              }
              n669 = Divide(x=w1448, y=w1445) -> (x/y=w1452:dbl[])
              n670 = local read "Output Directory"() -> (w1461:path)
              n671 = local read "df XPS"() -> (w1444:dbl)
              n672 = case shown="True" w1443 {
                tunnel: w1445 -> [w1477 _]
                tunnel: [w1477 w1479] -> w1446
                tunnel: w1444 -> [_ w1480]
                tunnel: w1447 -> [_ w1478]
                frame False {
                }
                frame True {
                  n673 = Add Array Elements(numeric array=w1478) -> (sum=w1481:dbl)
                  n674 = Multiply(x=w1481, y=w1480) -> (x*y=w1479:dbl)
                }
              }
              n675 = Divide(x=w1447, y=w1446) -> (x/y=w1454:dbl[])
              n676 = Array Size(array=w1447) -> (size(s)=w1451:i32)
              n677 = local read "Output Directory"() -> (w1468:path)
              n678 = Concatenate Strings(w1427, w1459) -> (w1462:string)
              n679 = expression code="0.5*df"(w1444) -> (w1450:dbl)
              n680 = Build Path(base path=w1461, name or relative path=w1462) -> (appended path=w1460:path)
              n681 = Concatenate Strings(w1429, w1459) -> (w1467:string)
              n682 = for {
                N: w1451 -> [_]
                shift-right: [w1484] -> _
                shift-left: w1450 -> [w1482]
                tunnel: w1444 -> [w1483]
                tunnel: [w1482] -> w1453 mode=indexing
                n683 = Add(x=w1482, y=w1483) -> (x+y=w1484:dbl)
              }
              n684 = Build Array(w1453, w1454) -> (w1464:dbl[][])
              n685 = Build Array(w1453, w1452) -> (w1457:dbl[][])
              n686 = Transpose 2D Array(2D array=w1464) -> (transposed array=w1463:dbl[][])
              n687 = Transpose 2D Array(2D array=w1457) -> (transposed array=w1458:dbl[][])
              n688 = Array To Spreadsheet String(array=w1463, 3:w1456) -> (spreadsheet string=w1438:string)  [unwired: 1 out]
              n689 = Array To Spreadsheet String(array=w1458, 3:w1456) -> (spreadsheet string=w1432:string)  [unwired: 1 out]
              n690 = Build Path(base path=w1468, name or relative path=w1467) -> (appended path=w1465:path)
              n691 = Format Into String(initial string="f (Hz)" ("string"), "\t", w1428, "\r", w1438) -> (resulting string=w1439:string)  [unwired: 2 in, 1 out]
              n692 = Format Into String(initial string="f (Hz)" ("string"), "\t", "Phi (deg)" ("string"), "\r", w1432) -> (resulting string=w1433:string)  [unwired: 2 in, 1 out]
              n693 = Write to Text File(file (use dialog)=w1465, text=w1439) -> ()  [unwired: 1 in, 4 out]
              n694 = Write to Text File(file (use dialog)=w1460, text=w1433) -> ()  [unwired: 1 in, 4 out]
            }
            frame "D. Wavelet Xform (Morlet)" {
            }
          }
        }
        "Plug in titles" <- w815
        "Plug in values" <- w814
      }
      frame "Create header string" {
        n695 = Strip Path(path=w1494) -> (stripped path=w1498:path, name=w1502:string)
        n696 = call "Remove_unprintable_Char.vi"("Input String"=w1502) -> ("Output String"=w1501:string)
        n697 = Path To String(path=w1498) -> (string=w1497:string)
        n698 = call "Characters_to_string.vi"("Characters to write"=w1501, "Label for characters"="Filename") -> ("Output string"=w1496:string)
        n699 = call "Remove_unprintable_Char.vi"("Input String"=w1497) -> ("Output String"=w1500:string)
        n700 = call "Value_to_string.vi"("Label for value"="LDA  Average Freq (Hz)") -> ("Output string"=w1505:string)  [unwired: 2 in]
        n701 = call "Characters_to_string.vi"("Characters to write"=w1500, "Label for characters"="File Path") -> ("Output string"=w1495:string)
        n702 = Concatenate Strings(w1496, w1495, w1505) -> (w1489:string)
      }
      frame "Full Header info" {
        w1510 = "\r"
        n703 = call "Read_RD_Ch_header.vi"("Raw data file"=w1507) -> ("Ch string"=w1508:string)  [unwired: 3 out]
        n704 = Concatenate Strings(w1513, w1510, "*****This is a many rows per single point file*****", w1510, w1508) -> (w1506:string)
      }
      frame "Add column titles" {
        w1522 = "\r"
        w1523 = "\r"
        n705 = case shown="\"Autocorrelation\"" w1531 {
          tunnel: ["f (Hz)" "Time (s)"] -> w1530
          tunnel: [" E(f)" " R(t,s)"] -> w1529
          frame "Spectra" {
          }
          frame "Autocorrelation" {
          }
        }
        n706 = local read "Ch names"() -> (w1536:string[])
        n707 = Initialize Array("", 10) -> (w1527:string[])
        n708 = call "Asterisk_header.vi"("Channel names"=w1527) -> ("Header string"=w1524:string)
        n709 = Concatenate Strings(w1528, w1522, w1524, w1522, w1522, w1530, "\t") -> (w1535:string)
        n710 = for {
          shift-right: [w1547] -> w1521
          shift-left: w1535 -> [w1549]
          tunnel: w1536 -> [w1550] mode=indexing
          tunnel: w1529 -> [w1546]
          n711 = Concatenate Strings(w1549, w1550, w1546, "\t") -> (w1547:string)
        }
        n712 = String Length(string=w1521) -> (length=w1518:i32)
        n713 = Decrement(x=w1518) -> (x-1=w1519:i32)
        n714 = String Subset(string=w1521, length (rest)=w1519) -> (substring=w1520:string)  [unwired: 1 out]
        n715 = Concatenate Strings(w1520, w1523, w1523) -> (w1534:string)
      }
      frame "Create Columns" {
        n716 = Array Size(array=w1557) -> (size(s)=w1555:i32[])
        n717 = Index Array(array=w1555, index=0) -> (element=w1554:i32)
        n718 = Decrement(x=w1554) -> (x-1=w1553:i32)
        n719 = for {
          shift-right: [w1580] -> w1561
          shift-left: "" -> [w1575]
          tunnel: "Separation Character" -> [w1568]
          tunnel: w1557 -> [w1578]
          tunnel: w1553 -> [w1574]
          tunnel: w1551 -> [w1572]
          tunnel: w1551 -> [w1571]
          tunnel: w1552 -> [w1567] mode=indexing
          i -> [w1573]
          n720 = Index Array(array=w1578, index (col)=w1573) -> (element=w1577:dbl[])  [unwired: 1 in]
          n721 = Number To Fractional String(number=w1567, precision (6)=w1571) -> (F-format string=w1570:string[])  [unwired: 2 out]
          n722 = Concatenate Strings(w1570, w1568) -> (w1569:string)
          n723 = for {
            shift-right: [w1587] -> w1576
            shift-left: w1569 -> [w1589]
            tunnel: w1568 -> [w1586]
            tunnel: w1577 -> [w1581] mode=indexing
            tunnel: w1574 -> [w1584]
            tunnel: w1572 -> [w1582]
            i -> [w1585]
            n724 = Equal?(x=w1585, y=w1584) -> (x = y?=w1583:bool)
            n725 = Number To Exponential String(number=w1581, precision (6)=w1582) -> (E-format string=w1588:string)  [unwired: 2 out]
            n726 = case shown="True" w1583 {
              tunnel: w1589 -> [w1593 w1596]
              tunnel: w1588 -> [w1592 w1595]
              tunnel: [w1591 w1594] -> w1587
              tunnel: w1586 -> [w1590 _]
              frame False {
                n727 = Concatenate Strings(w1593, w1592, w1590) -> (w1591:string)
              }
              frame True {
                n728 = Concatenate Strings(w1596, w1595) -> (w1594:string)
              }
            }
          }
          n729 = Concatenate Strings(w1575, w1576, "\r") -> (w1580:string)
        }
        n730 = Concatenate Strings(w1563, w1561) -> (w1562:string)
      }
      frame "Save to file" {
        w1603 = TRUE  # advisory dialog? (display:T)
        n731 = Strip Path(path=w1609) -> (name=w1607:string)  [unwired: 1 out]
        n732 = case shown="\"Autocorrelation\"" w1598 {
          tunnel: ["Spec_" ("string") "Auto_" ("string")] -> w1599
          frame "Spectra" {
          }
          frame "Autocorrelation" {
          }
        }
        n733 = local read "Output Directory"() -> (w1608:path)
        n734 = Concatenate Strings(w1599, w1607) -> (w1606:string)
        n735 = Build Path(base path=w1608, name or relative path=w1606) -> (appended path=w1605:path)
        n736 = call "Create_directory_path.vi"("Path name"=w1605) -> ("Path name Out"=w1604:path)
        n737 = call "Write_Characters_To_File.vi"("file path (dialog if empty)"=w1604, "advisory dialog? (display:T)"=w1603, "character string"=w1601, "append to file? (new file:F)"=FALSE) -> ()  [unwired: 1 in, 4 out]
      }
    }
  }
